vi "Measure vs B2Dv13.vi"() -> ()   [LabVIEW 2009]
doc: "This VI is an example operator panel.\n\nThe VI contains a table for the field values that may be configured manually, or loaded by checking the \"Prompt for File\" box. The data file should contain 3 columns of data, with each column delimited by a tab character.\n\nBefore the VI is executed, set the desired field units and coordinate system. Once the VI is started, follow the directions in the STATUS indicator to operate. Once a field value is achieved, it will be held indefinitely with no user intervention.\n\nThe present field is displayed in the selected units and coordinate system. The present field is queried once per second.\n\nIf a field point is specified that is outside the limits for the magnet, the VI will abort execution."
uses:
  <vilib>/Utility/file.llb/Read From Spreadsheet File (DBL).vi
panel:
  in  "TempSensor":bool
  in  "go to zero at end of measurement":bool=TRUE
  in  "AH (2500)":bool=TRUE
  out "fieldvalues":string[](array[string])
  in  "Nr. of Accumulations":i32=3
  out "appended array":dbl[](array[numeric])=[0.9997924469608681, 60.08772171794918, 0.0, 0.0, 0.0, 0.0, 0.0, 0.0, 0.0, 0.0, 0.0, 1.3266266666666666, -0.0011233333333333334, 0.0, 3432145944.794314]
  in  "X Axis":enum16{"B", "phi"}(ring)=enum."phi"
  in  "Y Axis":T1(ring)=enum."AH C (pF)"
  out "XY Graph":T2(graph)
  in  "GPIB HP 2":string="13"
  in  "Wait between \nVectors":bool=TRUE
  in  "Change\nPID\n(polar coordinates)":bool
  in  "Wait between \nVectors (ms)":u32=2000
  out "measured data":dbl[][](array[numeric])
  in  "Notes:":string="Datum: 3.10.12, Uhrzeit: 19:45, Sweep 0.15T/min,(measurevsB2Dv13.vi)), kapazitive Messung, Probe MnSi 10nm auf CuBe Cantilever (SI078)  tmeasure=ca. 4.3K,,   Einbauwinkel 15° (PraktikumsProbenstab) ,average time 3, winkelsweep mit0.5deg, Messbrücke auf Regal gestellt" caption="Notizen:"
  out "Messfile Refnum":refnum<file>
  in  "Measurement File":path=path "D:/UserData/Matthias/Messungen/MnSi/121003/SI078_121003_4K_m1.txt"
  in  "Sample name:":string="SI078"
  in  "HP 1":bool
  in  "GPIB HP":string="14"
  in  "HP 2":bool
  in  "LI 3":bool
  in  "GPIB L 3":string="8"
  in  "LI 2":bool
  in  "GPIB L 2":string="8"
  in  "LI 1":bool
  in  "GPIB L 1":string="8"
  out "Number of lines":i32=1804
  in  "Operation":u16(ring)=1 items=["Stepwise", "Continous"]
  out "Ramp Rate along Vector (T/min)":dbl=0.15 format="%.3f"
  out "Current Ramp Rate Z (T/min)":dbl=0.1299012842990965 format="%.3f"
  out "Current Ramp Rate Y (T/min)":dbl=0.07500437545533797 format="%.3f"
  in  "User defined Ramp Rate (T/min)":bool=TRUE
  in  "User defined Ramp Rate (T/min)":dbl=0.15 format="%.3f"
  in  "Z-Axis Communications Config":T3={"GPIB address"=22, "GPIB bus"=1, "connection ID"=refnum, "IP"="111.111.111.1", "Active Comm Interface"=0, "Serial Port"="", "Programmer Type"=0} {"Programmer Type" items=["Model 430", "Model 420"]; "Active Comm Interface" items=["TCP/IP (Model 430 Only)", "RS232", "IEEE488"]}
  in  "Max Ramp Rate - Y Axis (A/s)":dbl=0.055 format="%.3f"
  in  "Max Ramp Rate - Z Axis (A/s)":dbl=0.19 format="%.3f"
  in  "Magnitude Limit (kG)":dbl=45.1 format="%.3f"
  in  "Y-Axis Communications Config":T3={"GPIB address"=22, "GPIB bus"=1, "connection ID"=refnum, "IP"="111.111.111.2", "Active Comm Interface"=0, "Serial Port"="", "Programmer Type"=0} {"Programmer Type" items=["Model 430", "Model 420"]; "Active Comm Interface" items=["TCP/IP (Model 430 Only)", "RS232", "IEEE488"]}
  out "Cartesian Display (T)":T4={"Y-Axis Field (T)"=0.01746, "Z-Axis Field (T)"=0.99986} {"Z-Axis Field (T)" format="%.3f"; "Y-Axis Field (T)" format="%.3f"}
  in  "Starting index":i32=1804
  in  "Normal color":u32(colorbox)=11711154
  in  "Highlight color":u32(colorbox)=16711680
  in  "Prompt for File?":bool=TRUE
  out "Continue Execution?":bool
  out "error out":T5
  in  "error in":T5
  out "STATUS":string="Holding at current vector. Set Ramping Mode to NEXT VECTOR to continue."
  in  "Ramping Control":u16(ring)=2 items=["NEXT VECTOR", "RAMPING", "HOLDING", "PAUSE", "ZERO"]
  out "Cartesian Display (kG)":T6 {"Z-Axis Field (kG)" format="%.3f"; "Y-Axis Field (kG)" format="%.3f"}
  in  "Field Values":string[][](table)=[["0.0000", "60.0000"], ["0.3000", "60.0000"], ["0.3000", "60.5000"], ["0.3000", "61.0000"], ["0.3000", "61.5000"], ["0.3000", "62.0000"], ["0.3000", "62.5000"], ["0.3000", "63.0000"], ["0.3000", "63.5000"], ["0.3000", "64.0000"], ["0.3000", "64.5000"], ["0.3000", "65.0000"], ["0.3000", "65.5000"], ["0.3000", "66.0000"], ["0.3000", "66.5000"], ["0.3000", "67.0000"], ["0.3000", "67.5000"], ["0.3000", "68.0000"], ["0.3000", "68.5000"], ["0.3000", "69.0000"], ["0.3000", "69.5000"], ["0.3000", "70.0000"], ["0.3000", "70.5000"], ["0.3000", "71.0000"], ["0.3000", "71.5000"], ["0.3000", "72.0000"], ["0.3000", "72.5000"], ["0.3000", "73.0000"], ["0.3000", "73.5000"], ["0.3000", "74.0000"], ["0.3000", "74.5000"], ["0.3000", "75.0000"], ["0.3000", "75.5000"], ["0.3000", "76.0000"], ["0.3000", "76.5000"], ["0.3000", "77.0000"], ["0.3000", "77.5000"], ["0.3000", "78.0000"], ["0.3000", "78.5000"], ["0.3000", "79.0000"], ["0.3000", "79.5000"], ["0.3000", "80.0000"], ["0.3000", "80.5000"], ["0.3000", "81.0000"], ["0.3000", "81.5000"], ["0.3000", "82.0000"], ["0.3000", "82.5000"], ["0.3000", "83.0000"], ["0.3000", "83.5000"], ["0.3000", "84.0000"], ["0.3000", "84.5000"], ["0.3000", "85.0000"], ["0.3000", "85.5000"], ["0.3000", "86.0000"], ["0.3000", "86.5000"], ["0.3000", "87.0000"], ["0.3000", "87.5000"], ["0.3000", "88.0000"], ["0.3000", "88.5000"], ["0.3000", "89.0000"], ["0.3000", "89.5000"], ["0.3000", "90.0000"], ["0.3000", "90.5000"], ["0.3000", "91.0000"], ["0.3000", "91.5000"], ["0.3000", "92.0000"], ["0.3000", "92.5000"], ["0.3000", "93.0000"], ["0.3000", "93.5000"], ["0.3000", "94.0000"], ["0.3000", "94.5000"], ["0.3000", "95.0000"], ["0.3000", "95.5000"], ["0.3000", "96.0000"], ["0.3000", "96.5000"], ["0.3000", "97.0000"], ["0.3000", "97.5000"], ["0.3000", "98.0000"], ["0.3000", "98.5000"], ["0.3000", "99.0000"], ["0.3000", "99.5000"], ["0.3000", "100.0000"], ["0.3000", "100.5000"], ["0.3000", "101.0000"], ["0.3000", "101.5000"], ["0.3000", "102.0000"], ["0.3000", "102.5000"], ["0.3000", "103.0000"], ["0.3000", "103.5000"], ["0.3000", "104.0000"], ["0.3000", "104.5000"], ["0.3000", "105.0000"], ["0.3000", "105.5000"], ["0.3000", "106.0000"], ["0.3000", "106.5000"], ["0.3000", "107.0000"], ["0.3000", "107.5000"], ["0.3000", "108.0000"], ["0.3000", "108.5000"], ["0.3000", "109.0000"], ["0.3000", "109.5000"], ["0.3000", "110.0000"], ["0.3000", "110.5000"], ["0.3000", "111.0000"], ["0.3000", "111.5000"], ["0.3000", "112.0000"], ["0.3000", "112.5000"], ["0.3000", "113.0000"], ["0.3000", "113.5000"], ["0.3000", "114.0000"], ["0.3000", "114.5000"], ["0.3000", "115.0000"], ["0.3000", "115.5000"], ["0.3000", "116.0000"], ["0.3000", "116.5000"], ["0.3000", "117.0000"], ["0.3000", "117.5000"], ["0.3000", "118.0000"], ["0.3000", "118.5000"], ["0.3000", "119.0000"], ["0.3000", "119.5000"], ["0.3000", "120.0000"], ["0.3000", "120.5000"], ["0.3000", "121.0000"], ["0.3000", "121.5000"], ["0.3000", "122.0000"], ["0.3000", "122.5000"], ["0.3000", "123.0000"], ["0.3000", "123.5000"], ["0.3000", "124.0000"], ["0.3000", "124.5000"], ["0.3000", "125.0000"], ["0.3000", "125.5000"], ["0.3000", "126.0000"], ["0.3000", "126.5000"], ["0.3000", "127.0000"], ["0.3000", "127.5000"], ["0.3000", "128.0000"], ["0.3000", "128.5000"], ["0.3000", "129.0000"], ["0.3000", "129.5000"], ["0.3000", "130.0000"], ["0.3000", "130.5000"], ["0.3000", "131.0000"], ["0.3000", "131.5000"], ["0.3000", "132.0000"], ["0.3000", "132.5000"], ["0.3000", "133.0000"], ["0.3000", "133.5000"], ["0.3000", "134.0000"], ["0.3000", "134.5000"], ["0.3000", "135.0000"], ["0.3000", "135.5000"], ["0.3000", "136.0000"], ["0.3000", "136.5000"], ["0.3000", "137.0000"], ["0.3000", "137.5000"], ["0.3000", "138.0000"], ["0.3000", "138.5000"], ["0.3000", "139.0000"], ["0.3000", "139.5000"], ["0.3000", "140.0000"], ["0.3000", "140.5000"], ["0.3000", "141.0000"], ["0.3000", "141.5000"], ["0.3000", "142.0000"], ["0.3000", "142.5000"], ["0.3000", "143.0000"], ["0.3000", "143.5000"], ["0.3000", "144.0000"], ["0.3000", "144.5000"], ["0.3000", "145.0000"], ["0.3000", "145.5000"], ["0.3000", "146.0000"], ["0.3000", "146.5000"], ["0.3000", "147.0000"], ["0.3000", "147.5000"], ["0.3000", "148.0000"], ["0.3000", "148.5000"], ["0.3000", "149.0000"], ["0.3000", "149.5000"], ["0.3000", "150.0000"], ["0.3000", "150.5000"], ["0.3000", "151.0000"], ["0.3000", "151.5000"], ["0.3000", "152.0000"], ["0.3000", "152.5000"], ["0.3000", "153.0000"], ["0.3000", "153.5000"], ["0.3000", "154.0000"], ["0.3000", "154.5000"], ["0.3000", "155.0000"], ["0.3000", "155.5000"], ["0.3000", "156.0000"], ["0.3000", "156.5000"], ["0.3000", "157.0000"], ["0.3000", "157.5000"], ["0.3000", "158.0000"], ["0.3000", "158.5000"], ["0.3000", "159.0000"], ["0.3000", "159.5000"], ["0.3000", "160.0000"], ["0.3000", "160.5000"], ["0.3000", "161.0000"], ["0.3000", "161.5000"], ["0.3000", "162.0000"], ["0.3000", "162.5000"], ["0.3000", "163.0000"], ["0.3000", "163.5000"], ["0.3000", "164.0000"], ["0.3000", "164.5000"], ["0.3000", "165.0000"], ["0.3000", "165.5000"], ["0.3000", "166.0000"], ["0.3000", "166.5000"], ["0.3000", "167.0000"], ["0.3000", "167.5000"], ["0.3000", "168.0000"], ["0.3000", "168.5000"], ["0.3000", "169.0000"], ["0.3000", "169.5000"], ["0.3000", "170.0000"], ["0.3000", "170.5000"], ["0.3000", "171.0000"], ["0.3000", "171.5000"], ["0.3000", "172.0000"], ["0.3000", "172.5000"], ["0.3000", "173.0000"], ["0.3000", "173.5000"], ["0.3000", "174.0000"], ["0.3000", "174.5000"], ["0.3000", "175.0000"], ["0.3000", "175.5000"], ["0.3000", "176.0000"], ["0.3000", "176.5000"], ["0.3000", "177.0000"], ["0.3000", "177.5000"], ["0.3000", "178.0000"], ["0.3000", "178.5000"], ["0.3000", "179.0000"], ["0.3000", "179.5000"], ["0.3000", "180.0000"], ["0.3000", "180.5000"], ["0.3000", "181.0000"], ["0.3000", "181.5000"], ["0.3000", "182.0000"], ["0.3000", "182.5000"], ["0.3000", "183.0000"], ["0.3000", "183.5000"], ["0.3000", "184.0000"], ["0.3000", "184.5000"], ["0.3000", "185.0000"], ["0.3000", "185.5000"], ["0.3000", "186.0000"], ["0.3000", "186.5000"], ["0.3000", "187.0000"], ["0.3000", "187.5000"], ["0.3000", "188.0000"], ["0.3000", "188.5000"], ["0.3000", "189.0000"], ["0.3000", "189.5000"], ["0.3000", "190.0000"], ["0.3000", "190.5000"], ["0.3000", "191.0000"], ["0.3000", "191.5000"], ["0.3000", "192.0000"], ["0.3000", "192.5000"], ["0.3000", "193.0000"], ["0.3000", "193.5000"], ["0.3000", "194.0000"], ["0.3000", "194.5000"], ["0.3000", "195.0000"], ["0.3000", "195.5000"], ["0.3000", "196.0000"], ["0.3000", "196.5000"], ["0.3000", "197.0000"], ["0.3000", "197.5000"], ["0.3000", "198.0000"], ["0.3000", "198.5000"], ["0.3000", "199.0000"], ["0.3000", "199.5000"], ["0.3000", "200.0000"], ["0.3000", "200.5000"], ["0.3000", "201.0000"], ["0.3000", "201.5000"], ["0.3000", "202.0000"], ["0.3000", "202.5000"], ["0.3000", "203.0000"], ["0.3000", "203.5000"], ["0.3000", "204.0000"], ["0.3000", "204.5000"], ["0.3000", "205.0000"], ["0.3000", "205.5000"], ["0.3000", "206.0000"], ["0.3000", "206.5000"], ["0.3000", "207.0000"], ["0.3000", "207.5000"], ["0.3000", "208.0000"], ["0.3000", "208.5000"], ["0.3000", "209.0000"], ["0.3000", "209.5000"], ["0.3000", "210.0000"], ["0.3000", "210.5000"], ["0.3000", "211.0000"], ["0.3000", "211.5000"], ["0.3000", "212.0000"], ["0.3000", "212.5000"], ["0.3000", "213.0000"], ["0.3000", "213.5000"], ["0.3000", "214.0000"], ["0.3000", "214.5000"], ["0.3000", "215.0000"], ["0.3000", "215.5000"], ["0.3000", "216.0000"], ["0.3000", "216.5000"], ["0.3000", "217.0000"], ["0.3000", "217.5000"], ["0.3000", "218.0000"], ["0.3000", "218.5000"], ["0.3000", "219.0000"], ["0.3000", "219.5000"], ["0.3000", "220.0000"], ["0.3000", "220.5000"], ["0.3000", "221.0000"], ["0.3000", "221.5000"], ["0.3000", "222.0000"], ["0.3000", "222.5000"], ["0.3000", "223.0000"], ["0.3000", "223.5000"], ["0.3000", "224.0000"], ["0.3000", "224.5000"], ["0.3000", "225.0000"], ["0.3000", "225.5000"], ["0.3000", "226.0000"], ["0.3000", "226.5000"], ["0.3000", "227.0000"], ["0.3000", "227.5000"], ["0.3000", "228.0000"], ["0.3000", "228.5000"], ["0.3000", "229.0000"], ["0.3000", "229.5000"], ["0.3000", "230.0000"], ["0.3000", "230.5000"], ["0.3000", "231.0000"], ["0.3000", "231.5000"], ["0.3000", "232.0000"], ["0.3000", "232.5000"], ["0.3000", "233.0000"], ["0.3000", "233.5000"], ["0.3000", "234.0000"], ["0.3000", "234.5000"], ["0.3000", "235.0000"], ["0.3000", "235.5000"], ["0.3000", "236.0000"], ["0.3000", "236.5000"], ["0.3000", "237.0000"], ["0.3000", "237.5000"], ["0.3000", "238.0000"], ["0.3000", "238.5000"], ["0.3000", "239.0000"], ["0.3000", "239.5000"], ["0.3000", "240.0000"], ["0.3000", "240.5000"], ["0.3000", "241.0000"], ["0.3000", "241.5000"], ["0.3000", "242.0000"], ["0.3000", "242.5000"], ["0.3000", "243.0000"], ["0.3000", "243.5000"], ["0.3000", "244.0000"], ["0.3000", "244.5000"], ["0.3000", "245.0000"], ["0.3000", "245.5000"], ["0.3000", "246.0000"], ["0.3000", "246.5000"], ["0.3000", "247.0000"], ["0.3000", "247.5000"], ["0.3000", "248.0000"], ["0.3000", "248.5000"], ["0.3000", "249.0000"], ["0.3000", "249.5000"], ["0.3000", "250.0000"], ["0.3000", "250.5000"], ["0.3000", "251.0000"], ["0.3000", "251.5000"], ["0.3000", "252.0000"], ["0.3000", "252.5000"], ["0.3000", "253.0000"], ["0.3000", "253.5000"], ["0.3000", "254.0000"], ["0.3000", "254.5000"], ["0.3000", "255.0000"], ["0.3000", "255.5000"], ["0.3000", "256.0000"], ["0.3000", "256.5000"], ["0.3000", "257.0000"], ["0.3000", "257.5000"], ["0.3000", "258.0000"], ["0.3000", "258.5000"], ["0.3000", "259.0000"], ["0.3000", "259.5000"], ["0.3000", "260.0000"], ["0.3000", "260.5000"], ["0.3000", "261.0000"], ["0.3000", "261.5000"], ["0.3000", "262.0000"], ["0.3000", "262.5000"], ["0.3000", "263.0000"], ["0.3000", "263.5000"], ["0.3000", "264.0000"], ["0.3000", "264.5000"], ["0.3000", "265.0000"], ["0.3000", "265.5000"], ["0.3000", "266.0000"], ["0.3000", "266.5000"], ["0.3000", "267.0000"], ["0.3000", "267.5000"], ["0.3000", "268.0000"], ["0.3000", "268.5000"], ["0.3000", "269.0000"], ["0.3000", "269.5000"], ["0.3000", "270.0000"], ["0.3000", "270.5000"], ["0.3000", "271.0000"], ["0.3000", "271.5000"], ["0.3000", "272.0000"], ["0.3000", "272.5000"], ["0.3000", "273.0000"], ["0.3000", "273.5000"], ["0.3000", "274.0000"], ["0.3000", "274.5000"], ["0.3000", "275.0000"], ["0.3000", "275.5000"], ["0.3000", "276.0000"], ["0.3000", "276.5000"], ["0.3000", "277.0000"], ["0.3000", "277.5000"], ["0.3000", "278.0000"], ["0.3000", "278.5000"], ["0.3000", "279.0000"], ["0.3000", "279.5000"], ["0.3000", "280.0000"], ["0.3000", "280.5000"], ["0.3000", "281.0000"], ["0.3000", "281.5000"], ["0.3000", "282.0000"], ["0.3000", "282.5000"], ["0.3000", "283.0000"], ["0.3000", "283.5000"], ["0.3000", "284.0000"], ["0.3000", "284.5000"], ["0.3000", "285.0000"], ["0.3000", "284.5000"], ["0.3000", "284.0000"], ["0.3000", "283.5000"], ["0.3000", "283.0000"], ["0.3000", "282.5000"], ["0.3000", "282.0000"], ["0.3000", "281.5000"], ["0.3000", "281.0000"], ["0.3000", "280.5000"], ["0.3000", "280.0000"], ["0.3000", "279.5000"], ["0.3000", "279.0000"], ["0.3000", "278.5000"], ["0.3000", "278.0000"], ["0.3000", "277.5000"], ["0.3000", "277.0000"], ["0.3000", "276.5000"], ["0.3000", "276.0000"], ["0.3000", "275.5000"], ["0.3000", "275.0000"], ["0.3000", "274.5000"], ["0.3000", "274.0000"], ["0.3000", "273.5000"], ["0.3000", "273.0000"], ["0.3000", "272.5000"], ["0.3000", "272.0000"], ["0.3000", "271.5000"], ["0.3000", "271.0000"], ["0.3000", "270.5000"], ["0.3000", "270.0000"], ["0.3000", "269.5000"], ["0.3000", "269.0000"], ["0.3000", "268.5000"], ["0.3000", "268.0000"], ["0.3000", "267.5000"], ["0.3000", "267.0000"], ["0.3000", "266.5000"], ["0.3000", "266.0000"], ["0.3000", "265.5000"], ["0.3000", "265.0000"], ["0.3000", "264.5000"], ["0.3000", "264.0000"], ["0.3000", "263.5000"], ["0.3000", "263.0000"], ["0.3000", "262.5000"], ["0.3000", "262.0000"], ["0.3000", "261.5000"], ["0.3000", "261.0000"], ["0.3000", "260.5000"], ["0.3000", "260.0000"], ["0.3000", "259.5000"], ["0.3000", "259.0000"], ["0.3000", "258.5000"], ["0.3000", "258.0000"], ["0.3000", "257.5000"], ["0.3000", "257.0000"], ["0.3000", "256.5000"], ["0.3000", "256.0000"], ["0.3000", "255.5000"], ["0.3000", "255.0000"], ["0.3000", "254.5000"], ["0.3000", "254.0000"], ["0.3000", "253.5000"], ["0.3000", "253.0000"], ["0.3000", "252.5000"], ["0.3000", "252.0000"], ["0.3000", "251.5000"], ["0.3000", "251.0000"], ["0.3000", "250.5000"], ["0.3000", "250.0000"], ["0.3000", "249.5000"], ["0.3000", "249.0000"], ["0.3000", "248.5000"], ["0.3000", "248.0000"], ["0.3000", "247.5000"], ["0.3000", "247.0000"], ["0.3000", "246.5000"], ["0.3000", "246.0000"], ["0.3000", "245.5000"], ["0.3000", "245.0000"], ["0.3000", "244.5000"], ["0.3000", "244.0000"], ["0.3000", "243.5000"], ["0.3000", "243.0000"], ["0.3000", "242.5000"], ["0.3000", "242.0000"], ["0.3000", "241.5000"], ["0.3000", "241.0000"], ["0.3000", "240.5000"], ["0.3000", "240.0000"], ["0.3000", "239.5000"], ["0.3000", "239.0000"], ["0.3000", "238.5000"], ["0.3000", "238.0000"], ["0.3000", "237.5000"], ["0.3000", "237.0000"], ["0.3000", "236.5000"], ["0.3000", "236.0000"], ["0.3000", "235.5000"], ["0.3000", "235.0000"], ["0.3000", "234.5000"], ["0.3000", "234.0000"], ["0.3000", "233.5000"], ["0.3000", "233.0000"], ["0.3000", "232.5000"], ["0.3000", "232.0000"], ["0.3000", "231.5000"], ["0.3000", "231.0000"], ["0.3000", "230.5000"], ["0.3000", "230.0000"], ["0.3000", "229.5000"], ["0.3000", "229.0000"], ["0.3000", "228.5000"], ["0.3000", "228.0000"], ["0.3000", "227.5000"], ["0.3000", "227.0000"], ["0.3000", "226.5000"], ["0.3000", "226.0000"], ["0.3000", "225.5000"], ["0.3000", "225.0000"], ["0.3000", "224.5000"], ["0.3000", "224.0000"], ["0.3000", "223.5000"], ["0.3000", "223.0000"], ["0.3000", "222.5000"], ["0.3000", "222.0000"], ["0.3000", "221.5000"], ["0.3000", "221.0000"], ["0.3000", "220.5000"], ["0.3000", "220.0000"], ["0.3000", "219.5000"], ["0.3000", "219.0000"], ["0.3000", "218.5000"], ["0.3000", "218.0000"], ["0.3000", "217.5000"], ["0.3000", "217.0000"], ["0.3000", "216.5000"], ["0.3000", "216.0000"], ["0.3000", "215.5000"], ["0.3000", "215.0000"], ["0.3000", "214.5000"], ["0.3000", "214.0000"], ["0.3000", "213.5000"], ["0.3000", "213.0000"], ["0.3000", "212.5000"], ["0.3000", "212.0000"], ["0.3000", "211.5000"], ["0.3000", "211.0000"], ["0.3000", "210.5000"], ["0.3000", "210.0000"], ["0.3000", "209.5000"], ["0.3000", "209.0000"], ["0.3000", "208.5000"], ["0.3000", "208.0000"], ["0.3000", "207.5000"], ["0.3000", "207.0000"], ["0.3000", "206.5000"], ["0.3000", "206.0000"], ["0.3000", "205.5000"], ["0.3000", "205.0000"], ["0.3000", "204.5000"], ["0.3000", "204.0000"], ["0.3000", "203.5000"], ["0.3000", "203.0000"], ["0.3000", "202.5000"], ["0.3000", "202.0000"], ["0.3000", "201.5000"], ["0.3000", "201.0000"], ["0.3000", "200.5000"], ["0.3000", "200.0000"], ["0.3000", "199.5000"], ["0.3000", "199.0000"], ["0.3000", "198.5000"], ["0.3000", "198.0000"], ["0.3000", "197.5000"], ["0.3000", "197.0000"], ["0.3000", "196.5000"], ["0.3000", "196.0000"], ["0.3000", "195.5000"], ["0.3000", "195.0000"], ["0.3000", "194.5000"], ["0.3000", "194.0000"], ["0.3000", "193.5000"], ["0.3000", "193.0000"], ["0.3000", "192.5000"], ["0.3000", "192.0000"], ["0.3000", "191.5000"], ["0.3000", "191.0000"], ["0.3000", "190.5000"], ["0.3000", "190.0000"], ["0.3000", "189.5000"], ["0.3000", "189.0000"], ["0.3000", "188.5000"], ["0.3000", "188.0000"], ["0.3000", "187.5000"], ["0.3000", "187.0000"], ["0.3000", "186.5000"], ["0.3000", "186.0000"], ["0.3000", "185.5000"], ["0.3000", "185.0000"], ["0.3000", "184.5000"], ["0.3000", "184.0000"], ["0.3000", "183.5000"], ["0.3000", "183.0000"], ["0.3000", "182.5000"], ["0.3000", "182.0000"], ["0.3000", "181.5000"], ["0.3000", "181.0000"], ["0.3000", "180.5000"], ["0.3000", "180.0000"], ["0.3000", "179.5000"], ["0.3000", "179.0000"], ["0.3000", "178.5000"], ["0.3000", "178.0000"], ["0.3000", "177.5000"], ["0.3000", "177.0000"], ["0.3000", "176.5000"], ["0.3000", "176.0000"], ["0.3000", "175.5000"], ["0.3000", "175.0000"], ["0.3000", "174.5000"], ["0.3000", "174.0000"], ["0.3000", "173.5000"], ["0.3000", "173.0000"], ["0.3000", "172.5000"], ["0.3000", "172.0000"], ["0.3000", "171.5000"], ["0.3000", "171.0000"], ["0.3000", "170.5000"], ["0.3000", "170.0000"], ["0.3000", "169.5000"], ["0.3000", "169.0000"], ["0.3000", "168.5000"], ["0.3000", "168.0000"], ["0.3000", "167.5000"], ["0.3000", "167.0000"], ["0.3000", "166.5000"], ["0.3000", "166.0000"], ["0.3000", "165.5000"], ["0.3000", "165.0000"], ["0.3000", "164.5000"], ["0.3000", "164.0000"], ["0.3000", "163.5000"], ["0.3000", "163.0000"], ["0.3000", "162.5000"], ["0.3000", "162.0000"], ["0.3000", "161.5000"], ["0.3000", "161.0000"], ["0.3000", "160.5000"], ["0.3000", "160.0000"], ["0.3000", "159.5000"], ["0.3000", "159.0000"], ["0.3000", "158.5000"], ["0.3000", "158.0000"], ["0.3000", "157.5000"], ["0.3000", "157.0000"], ["0.3000", "156.5000"], ["0.3000", "156.0000"], ["0.3000", "155.5000"], ["0.3000", "155.0000"], ["0.3000", "154.5000"], ["0.3000", "154.0000"], ["0.3000", "153.5000"], ["0.3000", "153.0000"], ["0.3000", "152.5000"], ["0.3000", "152.0000"], ["0.3000", "151.5000"], ["0.3000", "151.0000"], ["0.3000", "150.5000"], ["0.3000", "150.0000"], ["0.3000", "149.5000"], ["0.3000", "149.0000"], ["0.3000", "148.5000"], ["0.3000", "148.0000"], ["0.3000", "147.5000"], ["0.3000", "147.0000"], ["0.3000", "146.5000"], ["0.3000", "146.0000"], ["0.3000", "145.5000"], ["0.3000", "145.0000"], ["0.3000", "144.5000"], ["0.3000", "144.0000"], ["0.3000", "143.5000"], ["0.3000", "143.0000"], ["0.3000", "142.5000"], ["0.3000", "142.0000"], ["0.3000", "141.5000"], ["0.3000", "141.0000"], ["0.3000", "140.5000"], ["0.3000", "140.0000"], ["0.3000", "139.5000"], ["0.3000", "139.0000"], ["0.3000", "138.5000"], ["0.3000", "138.0000"], ["0.3000", "137.5000"], ["0.3000", "137.0000"], ["0.3000", "136.5000"], ["0.3000", "136.0000"], ["0.3000", "135.5000"], ["0.3000", "135.0000"], ["0.3000", "134.5000"], ["0.3000", "134.0000"], ["0.3000", "133.5000"], ["0.3000", "133.0000"], ["0.3000", "132.5000"], ["0.3000", "132.0000"], ["0.3000", "131.5000"], ["0.3000", "131.0000"], ["0.3000", "130.5000"], ["0.3000", "130.0000"], ["0.3000", "129.5000"], ["0.3000", "129.0000"], ["0.3000", "128.5000"], ["0.3000", "128.0000"], ["0.3000", "127.5000"], ["0.3000", "127.0000"], ["0.3000", "126.5000"], ["0.3000", "126.0000"], ["0.3000", "125.5000"], ["0.3000", "125.0000"], ["0.3000", "124.5000"], ["0.3000", "124.0000"], ["0.3000", "123.5000"], ["0.3000", "123.0000"], ["0.3000", "122.5000"], ["0.3000", "122.0000"], ["0.3000", "121.5000"], ["0.3000", "121.0000"], ["0.3000", "120.5000"], ["0.3000", "120.0000"], ["0.3000", "119.5000"], ["0.3000", "119.0000"], ["0.3000", "118.5000"], ["0.3000", "118.0000"], ["0.3000", "117.5000"], ["0.3000", "117.0000"], ["0.3000", "116.5000"], ["0.3000", "116.0000"], ["0.3000", "115.5000"], ["0.3000", "115.0000"], ["0.3000", "114.5000"], ["0.3000", "114.0000"], ["0.3000", "113.5000"], ["0.3000", "113.0000"], ["0.3000", "112.5000"], ["0.3000", "112.0000"], ["0.3000", "111.5000"], ["0.3000", "111.0000"], ["0.3000", "110.5000"], ["0.3000", "110.0000"], ["0.3000", "109.5000"], ["0.3000", "109.0000"], ["0.3000", "108.5000"], ["0.3000", "108.0000"], ["0.3000", "107.5000"], ["0.3000", "107.0000"], ["0.3000", "106.5000"], ["0.3000", "106.0000"], ["0.3000", "105.5000"], ["0.3000", "105.0000"], ["0.3000", "104.5000"], ["0.3000", "104.0000"], ["0.3000", "103.5000"], ["0.3000", "103.0000"], ["0.3000", "102.5000"], ["0.3000", "102.0000"], ["0.3000", "101.5000"], ["0.3000", "101.0000"], ["0.3000", "100.5000"], ["0.3000", "100.0000"], ["0.3000", "99.5000"], ["0.3000", "99.0000"], ["0.3000", "98.5000"], ["0.3000", "98.0000"], ["0.3000", "97.5000"], ["0.3000", "97.0000"], ["0.3000", "96.5000"], ["0.3000", "96.0000"], ["0.3000", "95.5000"], ["0.3000", "95.0000"], ["0.3000", "94.5000"], ["0.3000", "94.0000"], ["0.3000", "93.5000"], ["0.3000", "93.0000"], ["0.3000", "92.5000"], ["0.3000", "92.0000"], ["0.3000", "91.5000"], ["0.3000", "91.0000"], ["0.3000", "90.5000"], ["0.3000", "90.0000"], ["0.3000", "89.5000"], ["0.3000", "89.0000"], ["0.3000", "88.5000"], ["0.3000", "88.0000"], ["0.3000", "87.5000"], ["0.3000", "87.0000"], ["0.3000", "86.5000"], ["0.3000", "86.0000"], ["0.3000", "85.5000"], ["0.3000", "85.0000"], ["0.3000", "84.5000"], ["0.3000", "84.0000"], ["0.3000", "83.5000"], ["0.3000", "83.0000"], ["0.3000", "82.5000"], ["0.3000", "82.0000"], ["0.3000", "81.5000"], ["0.3000", "81.0000"], ["0.3000", "80.5000"], ["0.3000", "80.0000"], ["0.3000", "79.5000"], ["0.3000", "79.0000"], ["0.3000", "78.5000"], ["0.3000", "78.0000"], ["0.3000", "77.5000"], ["0.3000", "77.0000"], ["0.3000", "76.5000"], ["0.3000", "76.0000"], ["0.3000", "75.5000"], ["0.3000", "75.0000"], ["0.3000", "74.5000"], ["0.3000", "74.0000"], ["0.3000", "73.5000"], ["0.3000", "73.0000"], ["0.3000", "72.5000"], ["0.3000", "72.0000"], ["0.3000", "71.5000"], ["0.3000", "71.0000"], ["0.3000", "70.5000"], ["0.3000", "70.0000"], ["0.3000", "69.5000"], ["0.3000", "69.0000"], ["0.3000", "68.5000"], ["0.3000", "68.0000"], ["0.3000", "67.5000"], ["0.3000", "67.0000"], ["0.3000", "66.5000"], ["0.3000", "66.0000"], ["0.3000", "65.5000"], ["0.3000", "65.0000"], ["0.3000", "64.5000"], ["0.3000", "64.0000"], ["0.3000", "63.5000"], ["0.3000", "63.0000"], ["0.3000", "62.5000"], ["0.3000", "62.0000"], ["0.3000", "61.5000"], ["0.3000", "61.0000"], ["0.3000", "60.5000"], ["0.3000", "60.0000"], ["1.0000", "60.0000"], ["1.0000", "60.5000"], ["1.0000", "61.0000"], ["1.0000", "61.5000"], ["1.0000", "62.0000"], ["1.0000", "62.5000"], ["1.0000", "63.0000"], ["1.0000", "63.5000"], ["1.0000", "64.0000"], ["1.0000", "64.5000"], ["1.0000", "65.0000"], ["1.0000", "65.5000"], ["1.0000", "66.0000"], ["1.0000", "66.5000"], ["1.0000", "67.0000"], ["1.0000", "67.5000"], ["1.0000", "68.0000"], ["1.0000", "68.5000"], ["1.0000", "69.0000"], ["1.0000", "69.5000"], ["1.0000", "70.0000"], ["1.0000", "70.5000"], ["1.0000", "71.0000"], ["1.0000", "71.5000"], ["1.0000", "72.0000"], ["1.0000", "72.5000"], ["1.0000", "73.0000"], ["1.0000", "73.5000"], ["1.0000", "74.0000"], ["1.0000", "74.5000"], ["1.0000", "75.0000"], ["1.0000", "75.5000"], ["1.0000", "76.0000"], ["1.0000", "76.5000"], ["1.0000", "77.0000"], ["1.0000", "77.5000"], ["1.0000", "78.0000"], ["1.0000", "78.5000"], ["1.0000", "79.0000"], ["1.0000", "79.5000"], ["1.0000", "80.0000"], ["1.0000", "80.5000"], ["1.0000", "81.0000"], ["1.0000", "81.5000"], ["1.0000", "82.0000"], ["1.0000", "82.5000"], ["1.0000", "83.0000"], ["1.0000", "83.5000"], ["1.0000", "84.0000"], ["1.0000", "84.5000"], ["1.0000", "85.0000"], ["1.0000", "85.5000"], ["1.0000", "86.0000"], ["1.0000", "86.5000"], ["1.0000", "87.0000"], ["1.0000", "87.5000"], ["1.0000", "88.0000"], ["1.0000", "88.5000"], ["1.0000", "89.0000"], ["1.0000", "89.5000"], ["1.0000", "90.0000"], ["1.0000", "90.5000"], ["1.0000", "91.0000"], ["1.0000", "91.5000"], ["1.0000", "92.0000"], ["1.0000", "92.5000"], ["1.0000", "93.0000"], ["1.0000", "93.5000"], ["1.0000", "94.0000"], ["1.0000", "94.5000"], ["1.0000", "95.0000"], ["1.0000", "95.5000"], ["1.0000", "96.0000"], ["1.0000", "96.5000"], ["1.0000", "97.0000"], ["1.0000", "97.5000"], ["1.0000", "98.0000"], ["1.0000", "98.5000"], ["1.0000", "99.0000"], ["1.0000", "99.5000"], ["1.0000", "100.0000"], ["1.0000", "100.5000"], ["1.0000", "101.0000"], ["1.0000", "101.5000"], ["1.0000", "102.0000"], ["1.0000", "102.5000"], ["1.0000", "103.0000"], ["1.0000", "103.5000"], ["1.0000", "104.0000"], ["1.0000", "104.5000"], ["1.0000", "105.0000"], ["1.0000", "105.5000"], ["1.0000", "106.0000"], ["1.0000", "106.5000"], ["1.0000", "107.0000"], ["1.0000", "107.5000"], ["1.0000", "108.0000"], ["1.0000", "108.5000"], ["1.0000", "109.0000"], ["1.0000", "109.5000"], ["1.0000", "110.0000"], ["1.0000", "110.5000"], ["1.0000", "111.0000"], ["1.0000", "111.5000"], ["1.0000", "112.0000"], ["1.0000", "112.5000"], ["1.0000", "113.0000"], ["1.0000", "113.5000"], ["1.0000", "114.0000"], ["1.0000", "114.5000"], ["1.0000", "115.0000"], ["1.0000", "115.5000"], ["1.0000", "116.0000"], ["1.0000", "116.5000"], ["1.0000", "117.0000"], ["1.0000", "117.5000"], ["1.0000", "118.0000"], ["1.0000", "118.5000"], ["1.0000", "119.0000"], ["1.0000", "119.5000"], ["1.0000", "120.0000"], ["1.0000", "120.5000"], ["1.0000", "121.0000"], ["1.0000", "121.5000"], ["1.0000", "122.0000"], ["1.0000", "122.5000"], ["1.0000", "123.0000"], ["1.0000", "123.5000"], ["1.0000", "124.0000"], ["1.0000", "124.5000"], ["1.0000", "125.0000"], ["1.0000", "125.5000"], ["1.0000", "126.0000"], ["1.0000", "126.5000"], ["1.0000", "127.0000"], ["1.0000", "127.5000"], ["1.0000", "128.0000"], ["1.0000", "128.5000"], ["1.0000", "129.0000"], ["1.0000", "129.5000"], ["1.0000", "130.0000"], ["1.0000", "130.5000"], ["1.0000", "131.0000"], ["1.0000", "131.5000"], ["1.0000", "132.0000"], ["1.0000", "132.5000"], ["1.0000", "133.0000"], ["1.0000", "133.5000"], ["1.0000", "134.0000"], ["1.0000", "134.5000"], ["1.0000", "135.0000"], ["1.0000", "135.5000"], ["1.0000", "136.0000"], ["1.0000", "136.5000"], ["1.0000", "137.0000"], ["1.0000", "137.5000"], ["1.0000", "138.0000"], ["1.0000", "138.5000"], ["1.0000", "139.0000"], ["1.0000", "139.5000"], ["1.0000", "140.0000"], ["1.0000", "140.5000"], ["1.0000", "141.0000"], ["1.0000", "141.5000"], ["1.0000", "142.0000"], ["1.0000", "142.5000"], ["1.0000", "143.0000"], ["1.0000", "143.5000"], ["1.0000", "144.0000"], ["1.0000", "144.5000"], ["1.0000", "145.0000"], ["1.0000", "145.5000"], ["1.0000", "146.0000"], ["1.0000", "146.5000"], ["1.0000", "147.0000"], ["1.0000", "147.5000"], ["1.0000", "148.0000"], ["1.0000", "148.5000"], ["1.0000", "149.0000"], ["1.0000", "149.5000"], ["1.0000", "150.0000"], ["1.0000", "150.5000"], ["1.0000", "151.0000"], ["1.0000", "151.5000"], ["1.0000", "152.0000"], ["1.0000", "152.5000"], ["1.0000", "153.0000"], ["1.0000", "153.5000"], ["1.0000", "154.0000"], ["1.0000", "154.5000"], ["1.0000", "155.0000"], ["1.0000", "155.5000"], ["1.0000", "156.0000"], ["1.0000", "156.5000"], ["1.0000", "157.0000"], ["1.0000", "157.5000"], ["1.0000", "158.0000"], ["1.0000", "158.5000"], ["1.0000", "159.0000"], ["1.0000", "159.5000"], ["1.0000", "160.0000"], ["1.0000", "160.5000"], ["1.0000", "161.0000"], ["1.0000", "161.5000"], ["1.0000", "162.0000"], ["1.0000", "162.5000"], ["1.0000", "163.0000"], ["1.0000", "163.5000"], ["1.0000", "164.0000"], ["1.0000", "164.5000"], ["1.0000", "165.0000"], ["1.0000", "165.5000"], ["1.0000", "166.0000"], ["1.0000", "166.5000"], ["1.0000", "167.0000"], ["1.0000", "167.5000"], ["1.0000", "168.0000"], ["1.0000", "168.5000"], ["1.0000", "169.0000"], ["1.0000", "169.5000"], ["1.0000", "170.0000"], ["1.0000", "170.5000"], ["1.0000", "171.0000"], ["1.0000", "171.5000"], ["1.0000", "172.0000"], ["1.0000", "172.5000"], ["1.0000", "173.0000"], ["1.0000", "173.5000"], ["1.0000", "174.0000"], ["1.0000", "174.5000"], ["1.0000", "175.0000"], ["1.0000", "175.5000"], ["1.0000", "176.0000"], ["1.0000", "176.5000"], ["1.0000", "177.0000"], ["1.0000", "177.5000"], ["1.0000", "178.0000"], ["1.0000", "178.5000"], ["1.0000", "179.0000"], ["1.0000", "179.5000"], ["1.0000", "180.0000"], ["1.0000", "180.5000"], ["1.0000", "181.0000"], ["1.0000", "181.5000"], ["1.0000", "182.0000"], ["1.0000", "182.5000"], ["1.0000", "183.0000"], ["1.0000", "183.5000"], ["1.0000", "184.0000"], ["1.0000", "184.5000"], ["1.0000", "185.0000"], ["1.0000", "185.5000"], ["1.0000", "186.0000"], ["1.0000", "186.5000"], ["1.0000", "187.0000"], ["1.0000", "187.5000"], ["1.0000", "188.0000"], ["1.0000", "188.5000"], ["1.0000", "189.0000"], ["1.0000", "189.5000"], ["1.0000", "190.0000"], ["1.0000", "190.5000"], ["1.0000", "191.0000"], ["1.0000", "191.5000"], ["1.0000", "192.0000"], ["1.0000", "192.5000"], ["1.0000", "193.0000"], ["1.0000", "193.5000"], ["1.0000", "194.0000"], ["1.0000", "194.5000"], ["1.0000", "195.0000"], ["1.0000", "195.5000"], ["1.0000", "196.0000"], ["1.0000", "196.5000"], ["1.0000", "197.0000"], ["1.0000", "197.5000"], ["1.0000", "198.0000"], ["1.0000", "198.5000"], ["1.0000", "199.0000"], ["1.0000", "199.5000"], ["1.0000", "200.0000"], ["1.0000", "200.5000"], ["1.0000", "201.0000"], ["1.0000", "201.5000"], ["1.0000", "202.0000"], ["1.0000", "202.5000"], ["1.0000", "203.0000"], ["1.0000", "203.5000"], ["1.0000", "204.0000"], ["1.0000", "204.5000"], ["1.0000", "205.0000"], ["1.0000", "205.5000"], ["1.0000", "206.0000"], ["1.0000", "206.5000"], ["1.0000", "207.0000"], ["1.0000", "207.5000"], ["1.0000", "208.0000"], ["1.0000", "208.5000"], ["1.0000", "209.0000"], ["1.0000", "209.5000"], ["1.0000", "210.0000"], ["1.0000", "210.5000"], ["1.0000", "211.0000"], ["1.0000", "211.5000"], ["1.0000", "212.0000"], ["1.0000", "212.5000"], ["1.0000", "213.0000"], ["1.0000", "213.5000"], ["1.0000", "214.0000"], ["1.0000", "214.5000"], ["1.0000", "215.0000"], ["1.0000", "215.5000"], ["1.0000", "216.0000"], ["1.0000", "216.5000"], ["1.0000", "217.0000"], ["1.0000", "217.5000"], ["1.0000", "218.0000"], ["1.0000", "218.5000"], ["1.0000", "219.0000"], ["1.0000", "219.5000"], ["1.0000", "220.0000"], ["1.0000", "220.5000"], ["1.0000", "221.0000"], ["1.0000", "221.5000"], ["1.0000", "222.0000"], ["1.0000", "222.5000"], ["1.0000", "223.0000"], ["1.0000", "223.5000"], ["1.0000", "224.0000"], ["1.0000", "224.5000"], ["1.0000", "225.0000"], ["1.0000", "225.5000"], ["1.0000", "226.0000"], ["1.0000", "226.5000"], ["1.0000", "227.0000"], ["1.0000", "227.5000"], ["1.0000", "228.0000"], ["1.0000", "228.5000"], ["1.0000", "229.0000"], ["1.0000", "229.5000"], ["1.0000", "230.0000"], ["1.0000", "230.5000"], ["1.0000", "231.0000"], ["1.0000", "231.5000"], ["1.0000", "232.0000"], ["1.0000", "232.5000"], ["1.0000", "233.0000"], ["1.0000", "233.5000"], ["1.0000", "234.0000"], ["1.0000", "234.5000"], ["1.0000", "235.0000"], ["1.0000", "235.5000"], ["1.0000", "236.0000"], ["1.0000", "236.5000"], ["1.0000", "237.0000"], ["1.0000", "237.5000"], ["1.0000", "238.0000"], ["1.0000", "238.5000"], ["1.0000", "239.0000"], ["1.0000", "239.5000"], ["1.0000", "240.0000"], ["1.0000", "240.5000"], ["1.0000", "241.0000"], ["1.0000", "241.5000"], ["1.0000", "242.0000"], ["1.0000", "242.5000"], ["1.0000", "243.0000"], ["1.0000", "243.5000"], ["1.0000", "244.0000"], ["1.0000", "244.5000"], ["1.0000", "245.0000"], ["1.0000", "245.5000"], ["1.0000", "246.0000"], ["1.0000", "246.5000"], ["1.0000", "247.0000"], ["1.0000", "247.5000"], ["1.0000", "248.0000"], ["1.0000", "248.5000"], ["1.0000", "249.0000"], ["1.0000", "249.5000"], ["1.0000", "250.0000"], ["1.0000", "250.5000"], ["1.0000", "251.0000"], ["1.0000", "251.5000"], ["1.0000", "252.0000"], ["1.0000", "252.5000"], ["1.0000", "253.0000"], ["1.0000", "253.5000"], ["1.0000", "254.0000"], ["1.0000", "254.5000"], ["1.0000", "255.0000"], ["1.0000", "255.5000"], ["1.0000", "256.0000"], ["1.0000", "256.5000"], ["1.0000", "257.0000"], ["1.0000", "257.5000"], ["1.0000", "258.0000"], ["1.0000", "258.5000"], ["1.0000", "259.0000"], ["1.0000", "259.5000"], ["1.0000", "260.0000"], ["1.0000", "260.5000"], ["1.0000", "261.0000"], ["1.0000", "261.5000"], ["1.0000", "262.0000"], ["1.0000", "262.5000"], ["1.0000", "263.0000"], ["1.0000", "263.5000"], ["1.0000", "264.0000"], ["1.0000", "264.5000"], ["1.0000", "265.0000"], ["1.0000", "265.5000"], ["1.0000", "266.0000"], ["1.0000", "266.5000"], ["1.0000", "267.0000"], ["1.0000", "267.5000"], ["1.0000", "268.0000"], ["1.0000", "268.5000"], ["1.0000", "269.0000"], ["1.0000", "269.5000"], ["1.0000", "270.0000"], ["1.0000", "270.5000"], ["1.0000", "271.0000"], ["1.0000", "271.5000"], ["1.0000", "272.0000"], ["1.0000", "272.5000"], ["1.0000", "273.0000"], ["1.0000", "273.5000"], ["1.0000", "274.0000"], ["1.0000", "274.5000"], ["1.0000", "275.0000"], ["1.0000", "275.5000"], ["1.0000", "276.0000"], ["1.0000", "276.5000"], ["1.0000", "277.0000"], ["1.0000", "277.5000"], ["1.0000", "278.0000"], ["1.0000", "278.5000"], ["1.0000", "279.0000"], ["1.0000", "279.5000"], ["1.0000", "280.0000"], ["1.0000", "280.5000"], ["1.0000", "281.0000"], ["1.0000", "281.5000"], ["1.0000", "282.0000"], ["1.0000", "282.5000"], ["1.0000", "283.0000"], ["1.0000", "283.5000"], ["1.0000", "284.0000"], ["1.0000", "284.5000"], ["1.0000", "285.0000"], ["1.0000", "284.5000"], ["1.0000", "284.0000"], ["1.0000", "283.5000"], ["1.0000", "283.0000"], ["1.0000", "282.5000"], ["1.0000", "282.0000"], ["1.0000", "281.5000"], ["1.0000", "281.0000"], ["1.0000", "280.5000"], ["1.0000", "280.0000"], ["1.0000", "279.5000"], ["1.0000", "279.0000"], ["1.0000", "278.5000"], ["1.0000", "278.0000"], ["1.0000", "277.5000"], ["1.0000", "277.0000"], ["1.0000", "276.5000"], ["1.0000", "276.0000"], ["1.0000", "275.5000"], ["1.0000", "275.0000"], ["1.0000", "274.5000"], ["1.0000", "274.0000"], ["1.0000", "273.5000"], ["1.0000", "273.0000"], ["1.0000", "272.5000"], ["1.0000", "272.0000"], ["1.0000", "271.5000"], ["1.0000", "271.0000"], ["1.0000", "270.5000"], ["1.0000", "270.0000"], ["1.0000", "269.5000"], ["1.0000", "269.0000"], ["1.0000", "268.5000"], ["1.0000", "268.0000"], ["1.0000", "267.5000"], ["1.0000", "267.0000"], ["1.0000", "266.5000"], ["1.0000", "266.0000"], ["1.0000", "265.5000"], ["1.0000", "265.0000"], ["1.0000", "264.5000"], ["1.0000", "264.0000"], ["1.0000", "263.5000"], ["1.0000", "263.0000"], ["1.0000", "262.5000"], ["1.0000", "262.0000"], ["1.0000", "261.5000"], ["1.0000", "261.0000"], ["1.0000", "260.5000"], ["1.0000", "260.0000"], ["1.0000", "259.5000"], ["1.0000", "259.0000"], ["1.0000", "258.5000"], ["1.0000", "258.0000"], ["1.0000", "257.5000"], ["1.0000", "257.0000"], ["1.0000", "256.5000"], ["1.0000", "256.0000"], ["1.0000", "255.5000"], ["1.0000", "255.0000"], ["1.0000", "254.5000"], ["1.0000", "254.0000"], ["1.0000", "253.5000"], ["1.0000", "253.0000"], ["1.0000", "252.5000"], ["1.0000", "252.0000"], ["1.0000", "251.5000"], ["1.0000", "251.0000"], ["1.0000", "250.5000"], ["1.0000", "250.0000"], ["1.0000", "249.5000"], ["1.0000", "249.0000"], ["1.0000", "248.5000"], ["1.0000", "248.0000"], ["1.0000", "247.5000"], ["1.0000", "247.0000"], ["1.0000", "246.5000"], ["1.0000", "246.0000"], ["1.0000", "245.5000"], ["1.0000", "245.0000"], ["1.0000", "244.5000"], ["1.0000", "244.0000"], ["1.0000", "243.5000"], ["1.0000", "243.0000"], ["1.0000", "242.5000"], ["1.0000", "242.0000"], ["1.0000", "241.5000"], ["1.0000", "241.0000"], ["1.0000", "240.5000"], ["1.0000", "240.0000"], ["1.0000", "239.5000"], ["1.0000", "239.0000"], ["1.0000", "238.5000"], ["1.0000", "238.0000"], ["1.0000", "237.5000"], ["1.0000", "237.0000"], ["1.0000", "236.5000"], ["1.0000", "236.0000"], ["1.0000", "235.5000"], ["1.0000", "235.0000"], ["1.0000", "234.5000"], ["1.0000", "234.0000"], ["1.0000", "233.5000"], ["1.0000", "233.0000"], ["1.0000", "232.5000"], ["1.0000", "232.0000"], ["1.0000", "231.5000"], ["1.0000", "231.0000"], ["1.0000", "230.5000"], ["1.0000", "230.0000"], ["1.0000", "229.5000"], ["1.0000", "229.0000"], ["1.0000", "228.5000"], ["1.0000", "228.0000"], ["1.0000", "227.5000"], ["1.0000", "227.0000"], ["1.0000", "226.5000"], ["1.0000", "226.0000"], ["1.0000", "225.5000"], ["1.0000", "225.0000"], ["1.0000", "224.5000"], ["1.0000", "224.0000"], ["1.0000", "223.5000"], ["1.0000", "223.0000"], ["1.0000", "222.5000"], ["1.0000", "222.0000"], ["1.0000", "221.5000"], ["1.0000", "221.0000"], ["1.0000", "220.5000"], ["1.0000", "220.0000"], ["1.0000", "219.5000"], ["1.0000", "219.0000"], ["1.0000", "218.5000"], ["1.0000", "218.0000"], ["1.0000", "217.5000"], ["1.0000", "217.0000"], ["1.0000", "216.5000"], ["1.0000", "216.0000"], ["1.0000", "215.5000"], ["1.0000", "215.0000"], ["1.0000", "214.5000"], ["1.0000", "214.0000"], ["1.0000", "213.5000"], ["1.0000", "213.0000"], ["1.0000", "212.5000"], ["1.0000", "212.0000"], ["1.0000", "211.5000"], ["1.0000", "211.0000"], ["1.0000", "210.5000"], ["1.0000", "210.0000"], ["1.0000", "209.5000"], ["1.0000", "209.0000"], ["1.0000", "208.5000"], ["1.0000", "208.0000"], ["1.0000", "207.5000"], ["1.0000", "207.0000"], ["1.0000", "206.5000"], ["1.0000", "206.0000"], ["1.0000", "205.5000"], ["1.0000", "205.0000"], ["1.0000", "204.5000"], ["1.0000", "204.0000"], ["1.0000", "203.5000"], ["1.0000", "203.0000"], ["1.0000", "202.5000"], ["1.0000", "202.0000"], ["1.0000", "201.5000"], ["1.0000", "201.0000"], ["1.0000", "200.5000"], ["1.0000", "200.0000"], ["1.0000", "199.5000"], ["1.0000", "199.0000"], ["1.0000", "198.5000"], ["1.0000", "198.0000"], ["1.0000", "197.5000"], ["1.0000", "197.0000"], ["1.0000", "196.5000"], ["1.0000", "196.0000"], ["1.0000", "195.5000"], ["1.0000", "195.0000"], ["1.0000", "194.5000"], ["1.0000", "194.0000"], ["1.0000", "193.5000"], ["1.0000", "193.0000"], ["1.0000", "192.5000"], ["1.0000", "192.0000"], ["1.0000", "191.5000"], ["1.0000", "191.0000"], ["1.0000", "190.5000"], ["1.0000", "190.0000"], ["1.0000", "189.5000"], ["1.0000", "189.0000"], ["1.0000", "188.5000"], ["1.0000", "188.0000"], ["1.0000", "187.5000"], ["1.0000", "187.0000"], ["1.0000", "186.5000"], ["1.0000", "186.0000"], ["1.0000", "185.5000"], ["1.0000", "185.0000"], ["1.0000", "184.5000"], ["1.0000", "184.0000"], ["1.0000", "183.5000"], ["1.0000", "183.0000"], ["1.0000", "182.5000"], ["1.0000", "182.0000"], ["1.0000", "181.5000"], ["1.0000", "181.0000"], ["1.0000", "180.5000"], ["1.0000", "180.0000"], ["1.0000", "179.5000"], ["1.0000", "179.0000"], ["1.0000", "178.5000"], ["1.0000", "178.0000"], ["1.0000", "177.5000"], ["1.0000", "177.0000"], ["1.0000", "176.5000"], ["1.0000", "176.0000"], ["1.0000", "175.5000"], ["1.0000", "175.0000"], ["1.0000", "174.5000"], ["1.0000", "174.0000"], ["1.0000", "173.5000"], ["1.0000", "173.0000"], ["1.0000", "172.5000"], ["1.0000", "172.0000"], ["1.0000", "171.5000"], ["1.0000", "171.0000"], ["1.0000", "170.5000"], ["1.0000", "170.0000"], ["1.0000", "169.5000"], ["1.0000", "169.0000"], ["1.0000", "168.5000"], ["1.0000", "168.0000"], ["1.0000", "167.5000"], ["1.0000", "167.0000"], ["1.0000", "166.5000"], ["1.0000", "166.0000"], ["1.0000", "165.5000"], ["1.0000", "165.0000"], ["1.0000", "164.5000"], ["1.0000", "164.0000"], ["1.0000", "163.5000"], ["1.0000", "163.0000"], ["1.0000", "162.5000"], ["1.0000", "162.0000"], ["1.0000", "161.5000"], ["1.0000", "161.0000"], ["1.0000", "160.5000"], ["1.0000", "160.0000"], ["1.0000", "159.5000"], ["1.0000", "159.0000"], ["1.0000", "158.5000"], ["1.0000", "158.0000"], ["1.0000", "157.5000"], ["1.0000", "157.0000"], ["1.0000", "156.5000"], ["1.0000", "156.0000"], ["1.0000", "155.5000"], ["1.0000", "155.0000"], ["1.0000", "154.5000"], ["1.0000", "154.0000"], ["1.0000", "153.5000"], ["1.0000", "153.0000"], ["1.0000", "152.5000"], ["1.0000", "152.0000"], ["1.0000", "151.5000"], ["1.0000", "151.0000"], ["1.0000", "150.5000"], ["1.0000", "150.0000"], ["1.0000", "149.5000"], ["1.0000", "149.0000"], ["1.0000", "148.5000"], ["1.0000", "148.0000"], ["1.0000", "147.5000"], ["1.0000", "147.0000"], ["1.0000", "146.5000"], ["1.0000", "146.0000"], ["1.0000", "145.5000"], ["1.0000", "145.0000"], ["1.0000", "144.5000"], ["1.0000", "144.0000"], ["1.0000", "143.5000"], ["1.0000", "143.0000"], ["1.0000", "142.5000"], ["1.0000", "142.0000"], ["1.0000", "141.5000"], ["1.0000", "141.0000"], ["1.0000", "140.5000"], ["1.0000", "140.0000"], ["1.0000", "139.5000"], ["1.0000", "139.0000"], ["1.0000", "138.5000"], ["1.0000", "138.0000"], ["1.0000", "137.5000"], ["1.0000", "137.0000"], ["1.0000", "136.5000"], ["1.0000", "136.0000"], ["1.0000", "135.5000"], ["1.0000", "135.0000"], ["1.0000", "134.5000"], ["1.0000", "134.0000"], ["1.0000", "133.5000"], ["1.0000", "133.0000"], ["1.0000", "132.5000"], ["1.0000", "132.0000"], ["1.0000", "131.5000"], ["1.0000", "131.0000"], ["1.0000", "130.5000"], ["1.0000", "130.0000"], ["1.0000", "129.5000"], ["1.0000", "129.0000"], ["1.0000", "128.5000"], ["1.0000", "128.0000"], ["1.0000", "127.5000"], ["1.0000", "127.0000"], ["1.0000", "126.5000"], ["1.0000", "126.0000"], ["1.0000", "125.5000"], ["1.0000", "125.0000"], ["1.0000", "124.5000"], ["1.0000", "124.0000"], ["1.0000", "123.5000"], ["1.0000", "123.0000"], ["1.0000", "122.5000"], ["1.0000", "122.0000"], ["1.0000", "121.5000"], ["1.0000", "121.0000"], ["1.0000", "120.5000"], ["1.0000", "120.0000"], ["1.0000", "119.5000"], ["1.0000", "119.0000"], ["1.0000", "118.5000"], ["1.0000", "118.0000"], ["1.0000", "117.5000"], ["1.0000", "117.0000"], ["1.0000", "116.5000"], ["1.0000", "116.0000"], ["1.0000", "115.5000"], ["1.0000", "115.0000"], ["1.0000", "114.5000"], ["1.0000", "114.0000"], ["1.0000", "113.5000"], ["1.0000", "113.0000"], ["1.0000", "112.5000"], ["1.0000", "112.0000"], ["1.0000", "111.5000"], ["1.0000", "111.0000"], ["1.0000", "110.5000"], ["1.0000", "110.0000"], ["1.0000", "109.5000"], ["1.0000", "109.0000"], ["1.0000", "108.5000"], ["1.0000", "108.0000"], ["1.0000", "107.5000"], ["1.0000", "107.0000"], ["1.0000", "106.5000"], ["1.0000", "106.0000"], ["1.0000", "105.5000"], ["1.0000", "105.0000"], ["1.0000", "104.5000"], ["1.0000", "104.0000"], ["1.0000", "103.5000"], ["1.0000", "103.0000"], ["1.0000", "102.5000"], ["1.0000", "102.0000"], ["1.0000", "101.5000"], ["1.0000", "101.0000"], ["1.0000", "100.5000"], ["1.0000", "100.0000"], ["1.0000", "99.5000"], ["1.0000", "99.0000"], ["1.0000", "98.5000"], ["1.0000", "98.0000"], ["1.0000", "97.5000"], ["1.0000", "97.0000"], ["1.0000", "96.5000"], ["1.0000", "96.0000"], ["1.0000", "95.5000"], ["1.0000", "95.0000"], ["1.0000", "94.5000"], ["1.0000", "94.0000"], ["1.0000", "93.5000"], ["1.0000", "93.0000"], ["1.0000", "92.5000"], ["1.0000", "92.0000"], ["1.0000", "91.5000"], ["1.0000", "91.0000"], ["1.0000", "90.5000"], ["1.0000", "90.0000"], ["1.0000", "89.5000"], ["1.0000", "89.0000"], ["1.0000", "88.5000"], ["1.0000", "88.0000"], ["1.0000", "87.5000"], ["1.0000", "87.0000"], ["1.0000", "86.5000"], ["1.0000", "86.0000"], ["1.0000", "85.5000"], ["1.0000", "85.0000"], ["1.0000", "84.5000"], ["1.0000", "84.0000"], ["1.0000", "83.5000"], ["1.0000", "83.0000"], ["1.0000", "82.5000"], ["1.0000", "82.0000"], ["1.0000", "81.5000"], ["1.0000", "81.0000"], ["1.0000", "80.5000"], ["1.0000", "80.0000"], ["1.0000", "79.5000"], ["1.0000", "79.0000"], ["1.0000", "78.5000"], ["1.0000", "78.0000"], ["1.0000", "77.5000"], ["1.0000", "77.0000"], ["1.0000", "76.5000"], ["1.0000", "76.0000"], ["1.0000", "75.5000"], ["1.0000", "75.0000"], ["1.0000", "74.5000"], ["1.0000", "74.0000"], ["1.0000", "73.5000"], ["1.0000", "73.0000"], ["1.0000", "72.5000"], ["1.0000", "72.0000"], ["1.0000", "71.5000"], ["1.0000", "71.0000"], ["1.0000", "70.5000"], ["1.0000", "70.0000"], ["1.0000", "69.5000"], ["1.0000", "69.0000"], ["1.0000", "68.5000"], ["1.0000", "68.0000"], ["1.0000", "67.5000"], ["1.0000", "67.0000"], ["1.0000", "66.5000"], ["1.0000", "66.0000"], ["1.0000", "65.5000"], ["1.0000", "65.0000"], ["1.0000", "64.5000"], ["1.0000", "64.0000"], ["1.0000", "63.5000"], ["1.0000", "63.0000"], ["1.0000", "62.5000"], ["1.0000", "62.0000"], ["1.0000", "61.5000"], ["1.0000", "61.0000"], ["1.0000", "60.5000"], ["1.0000", "60.0000"], ["0.0000", "60.0000"]]
  out "Switch Heaters":bool=TRUE
  out "Polar Display (T)":T7={"q (degrees)"=59.03624346792648, "Field Magnitude (T)"=0.00011661903789690601} {"Field Magnitude (T)" format="%.3f"; "q (degrees)" format="%.3f"}
  out "Polar Display (kG)":T8 {"Field Magnitude (kG)" format="%.3f"; "q (degrees)" format="%.3f"}
  in  "Coordinate System":u16(ring)=1 items=["Cartesian", "Polar"]
  in  "Magnetic Field Units":u16(ring)=1 items=["kG", "Tesla"]
  # "Punkt für Punkt Messung, gotozero am Ende der Messung und switch heater off"
  # "Measurement Display"
  # "Measurement Settings"
  # "Magnet Settings"
  # "Max Ramp Rate z: 1.27 T/min\nMax Ramp Rate y: 0.17 T/min"
  # "Devices"
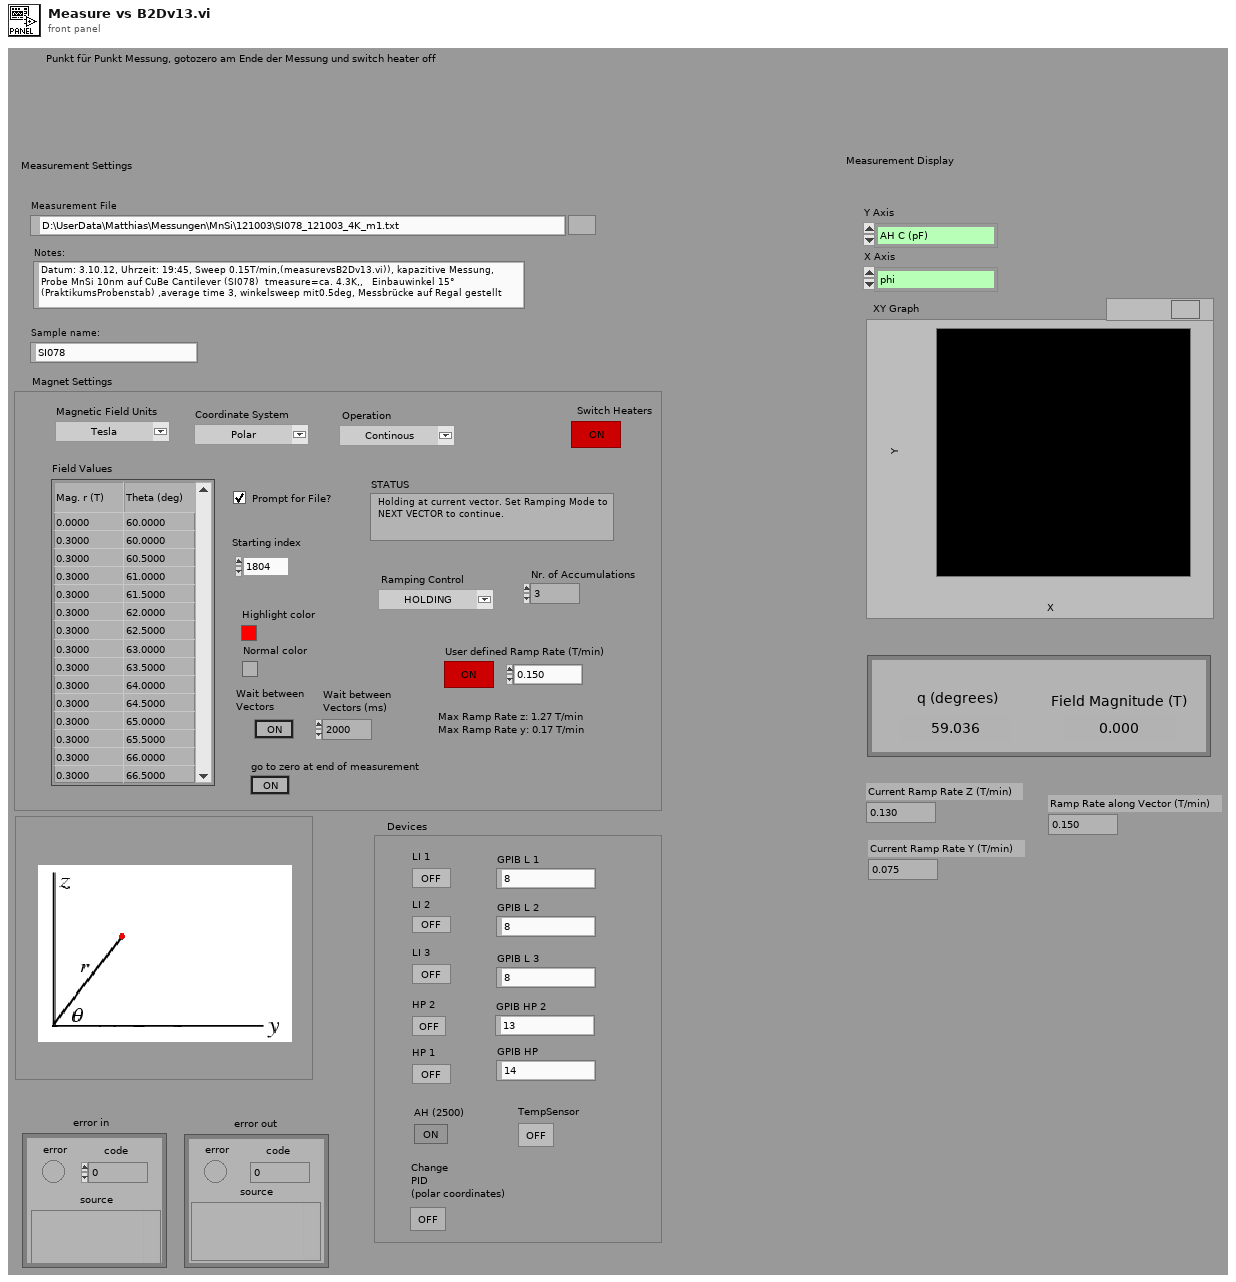
[diagram p1: front panel]
types:
  T1 = enum16{"B", "phi", "LI 1 Vx", "LI 1 phase", "LI 2 Vx", "LI 2 phase", "LI 3 Vx", "LI 3 phase", "LI 4 Vx", "LI 4 phase", "HP (V)", "AH C (pF)", "AH loss", "R Tempsensor"}
  T2 = cluster{"measured data":dbl[], "measured data":dbl[]}
  T3 = cluster{"GPIB address":i16, "GPIB bus":i16, "connection ID":refnum<k5>, "IP":string, "Active Comm Interface":u16, "Serial Port":refnum<visa-resource-name>, "Programmer Type":u16}
  T4 = cluster{"Y-Axis Field (T)":dbl, "Z-Axis Field (T)":dbl}
  T5 = cluster{"error":bool, "code":i32, "source":string}
  T6 = cluster{"Y-Axis Field (kG)":dbl, "Z-Axis Field (kG)":dbl}
  T7 = cluster{"q (degrees)":dbl, "Field Magnitude (T)":dbl}
  T8 = cluster{"q (degrees)":dbl, "Field Magnitude (kG)":dbl}
  T9 = enum16{"", "RAMPING", "HOLDING", "PAUSED", "MANUAL UP", "MANUAL DOWN", "ZEROING CURRENT", "QUENCH DETECTED", "HEATING SWITCH"}
  T10 = enum16{"", "RAMPING", "HOLDING", "PAUSED", "MANUAL UP", "MANUAL DOWN", "ZEROING CURRENT", "QUENCH DETECTED", "HEATING SWITCH", "AT ZER0", "COOLING SWITCH"}
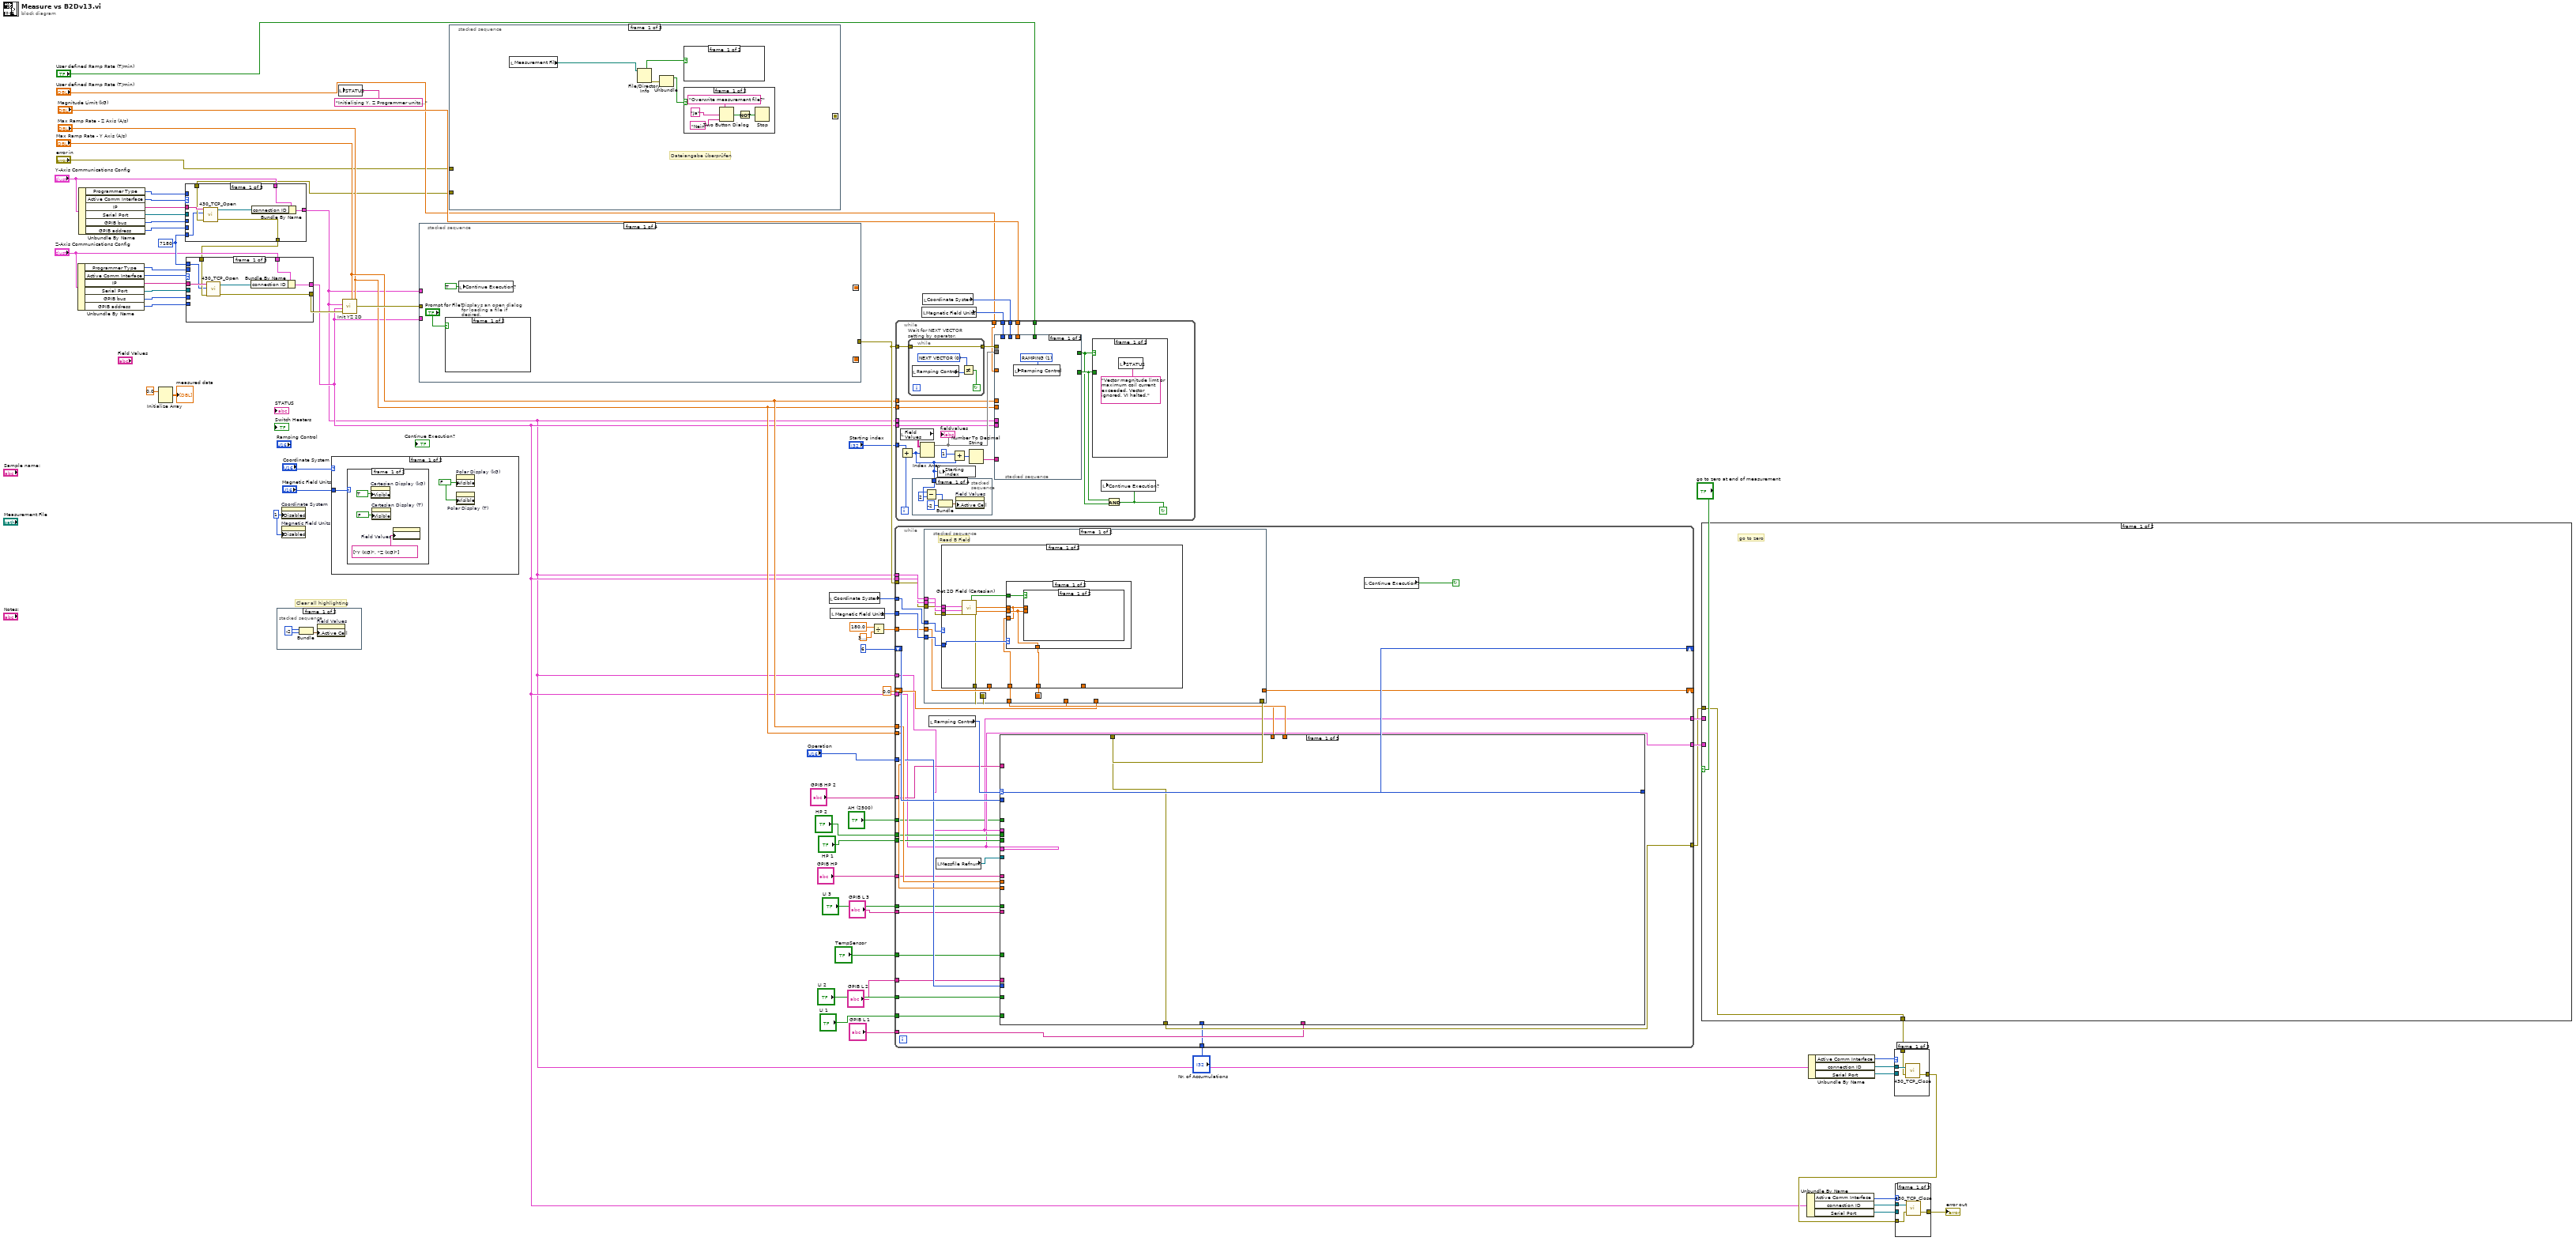
[diagram p0: block diagram]
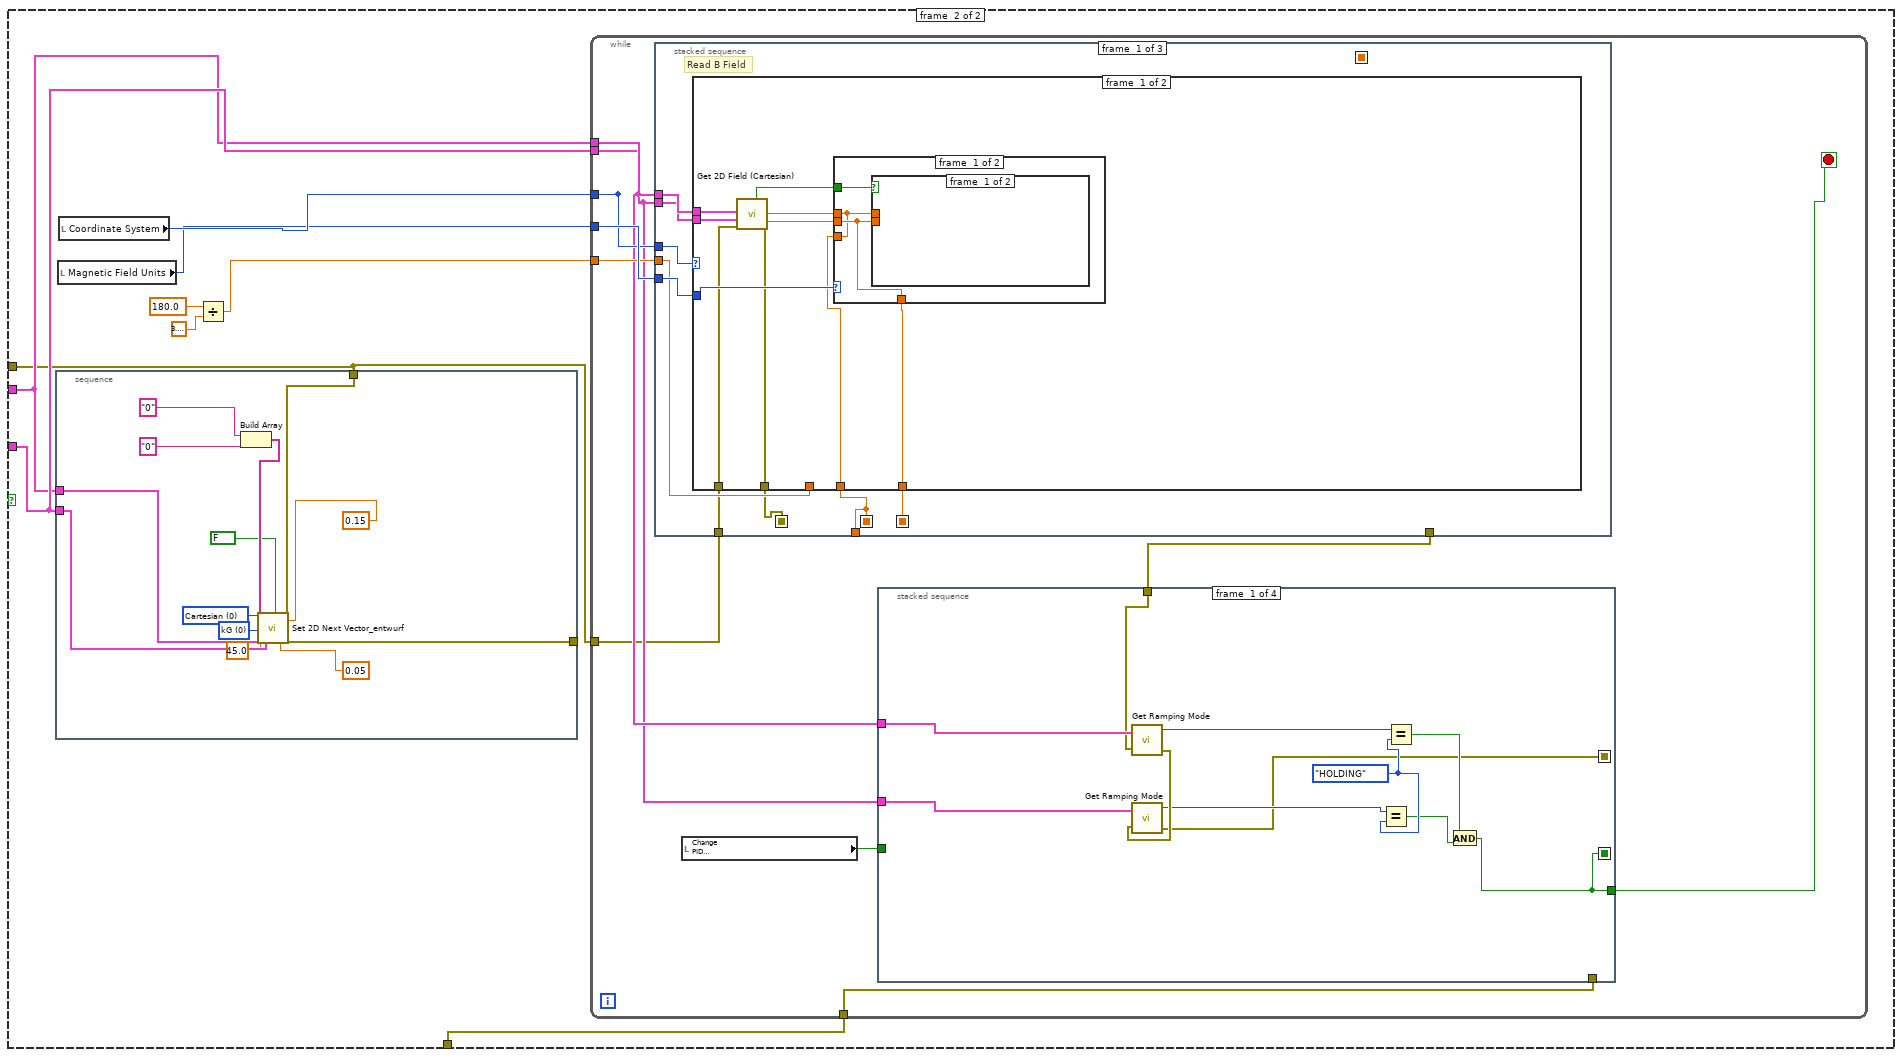
[diagram p2: hidden frame]
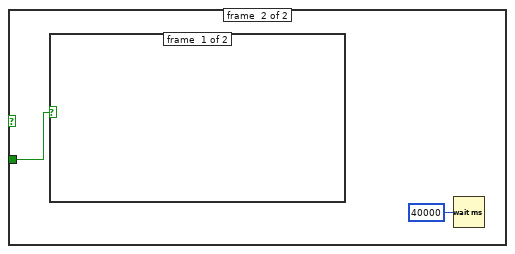
[diagram p4: hidden frame]
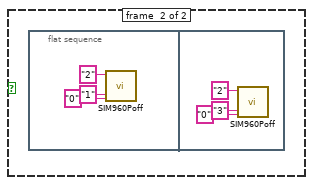
[diagram p5: hidden frame]
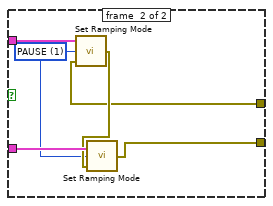
[diagram p7: hidden frame]
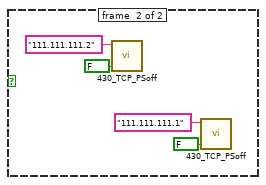
[diagram p9: hidden frame]
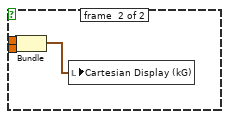
[diagram p10: hidden frame]
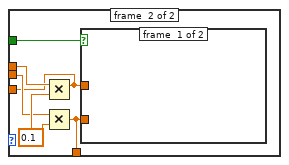
[diagram p11: hidden frame]
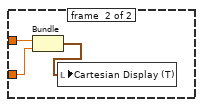
[diagram p12: hidden frame]
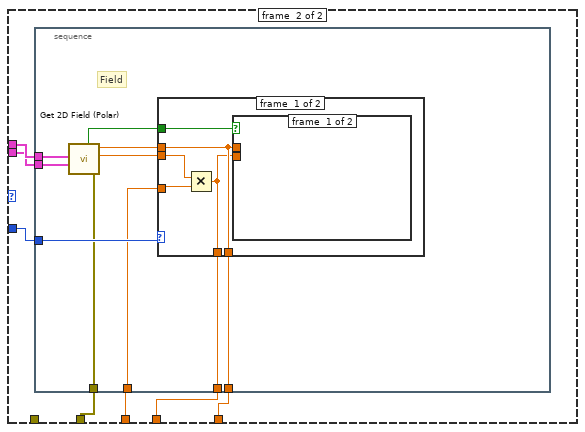
[diagram p13: hidden frame]
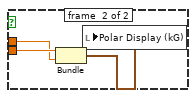
[diagram p14: hidden frame]
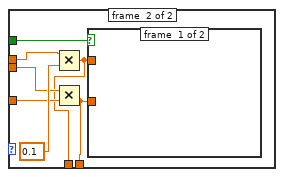
[diagram p15: hidden frame]
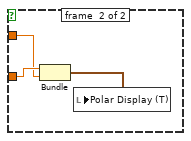
[diagram p16: hidden frame]
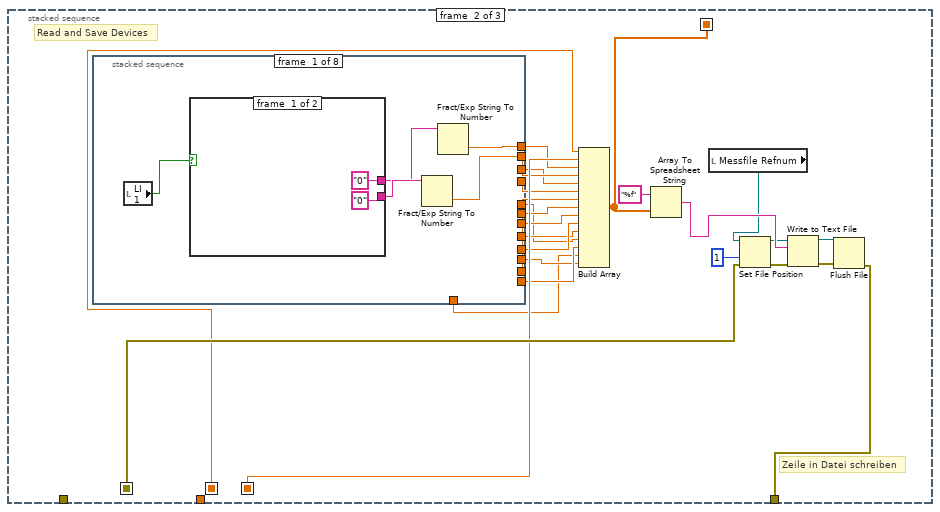
[diagram p17: hidden frame]
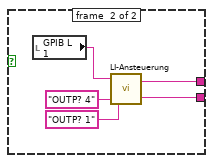
[diagram p18: hidden frame]
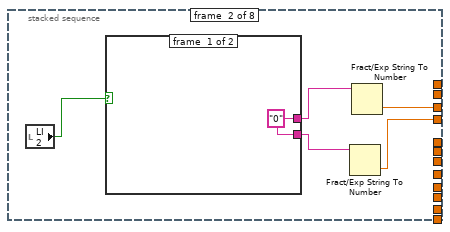
[diagram p19: hidden frame]
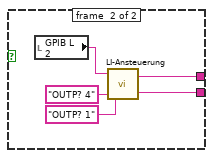
[diagram p20: hidden frame]
diagram:
  w56 = 7180 ("TCP Port")
  w69 = u8 1 ("Write Attribute")
  # "Clear all highlighting"
  n1 = Unbundle By Name("Z-Axis Communications Config") -> ("Programmer Type"=w35:u16, "Active Comm Interface"=w55:u16, "IP"=w52:string, "Serial Port"=w51:refnum<visa-resource-name>, "GPIB bus"=w34:i16, "GPIB address"=w33:i16)
  n2 = Unbundle By Name("Y-Axis Communications Config") -> ("Programmer Type"=w29:u16, "Active Comm Interface"=w54:u16, "IP"=w53:string, "Serial Port"=w50:refnum<visa-resource-name>, "GPIB bus"=w30:i16, "GPIB address"=w31:i16)
  n3 = Initialize Array(0.0 ("element")) -> (→"measured data":dbl[][])  [unwired: 2 in]
  n4 = stacked-sequence {
    frame #0 {
      w72 = -2
      n5 = Bundle(w72, w72) -> (w73:cluster{i32, i32})  [unwired: 1 in]
      n6 = property on="Field Values" class="Tbl (strict)"("Active Cell:Active Cell"=w73) -> ()  [unwired: 2 in, 2 out]
    }
    frame #1 {
      n7 = property on="Field Values" class="Tbl (strict)"("Active Cell:Cell Background Color"="Normal color") -> ()  [unwired: 2 in, 2 out]
    }
  }
  n8 = property on="Coordinate System" class="Ring (strict)"("Disabled"=w69) -> ()  [unwired: 2 in, 2 out]
  n9 = property on="Magnetic Field Units" class="Ring (strict)"("Disabled"=w69) -> ()  [unwired: 2 in, 2 out]
  n10 = case shown="0, Default" "Coordinate System" {
    tunnel: "Magnetic Field Units" -> [w76 w84]
    frame #0 {
      w75 = FALSE ("Write Attribute")
      (unwired) FALSE ("Write Attribute")
      (unwired) TRUE ("Write Attribute")
      n11 = case shown="1" w76 {
        frame #0 {
          n12 = property on="Cartesian Display (kG)" class="Cluster (strict)"("Visible"=TRUE ("Write Attribute")) -> ()  [unwired: 2 in, 2 out]
          n13 = property on="Cartesian Display (T)" class="Cluster (strict)"("Visible"=FALSE ("Write Attribute")) -> ()  [unwired: 2 in, 2 out]
          n14 = property on="Field Values" class="Tbl (strict)"("Column Header Strings[]"=string[] ["Y (KG)", "Z (KG)"] ("Write Attribute")) -> ()  [unwired: 2 in, 2 out]
        }
        frame #1 {
          n15 = property on="Cartesian Display (kG)" class="Cluster (strict)"("Visible"=FALSE ("Write Attribute")) -> ()  [unwired: 2 in, 2 out]
          n16 = property on="Cartesian Display (T)" class="Cluster (strict)"("Visible"=TRUE ("Write Attribute")) -> ()  [unwired: 2 in, 2 out]
          n17 = property on="Field Values" class="Tbl (strict)"("Column Header Strings[]"=string[] ["Y (T)", "Z (T)"] ("Write Attribute")) -> ()  [unwired: 2 in, 2 out]
        }
      }
      n18 = property on="Polar Display (kG)" class="Clust (strict)"("Visible"=w75) -> ()  [unwired: 2 in, 2 out]
      n19 = property on="Polar Display (T)" class="Clust (strict)"("Visible"=w75) -> ()  [unwired: 2 in, 2 out]
    }
    frame #1 {
      (unwired) FALSE ("Write Attribute")
      (unwired) TRUE ("Write Attribute")
      w83 = FALSE ("Write Attribute")
      n20 = case shown="1" w84 {
        frame #0 {
          n21 = property on="Polar Display (kG)" class="Clust (strict)"("Visible"=TRUE ("Write Attribute")) -> ()  [unwired: 2 in, 2 out]
          n22 = property on="Polar Display (T)" class="Clust (strict)"("Visible"=FALSE ("Write Attribute")) -> ()  [unwired: 2 in, 2 out]
          n23 = property on="Field Values" class="Tbl (strict)"("Column Header Strings[]"=string[] ["Mag. r (KG)", "Theta (deg)"] ("Write Attribute")) -> ()  [unwired: 2 in, 2 out]
        }
        frame #1 {
          n24 = property on="Polar Display (kG)" class="Clust (strict)"("Visible"=FALSE ("Write Attribute")) -> ()  [unwired: 2 in, 2 out]
          n25 = property on="Polar Display (T)" class="Clust (strict)"("Visible"=TRUE ("Write Attribute")) -> ()  [unwired: 2 in, 2 out]
          n26 = property on="Field Values" class="Tbl (strict)"("Column Header Strings[]"=string[] ["Mag. r (T)", "Theta (deg)"] ("Write Attribute")) -> ()  [unwired: 2 in, 2 out]
        }
      }
      n27 = property on="Cartesian Display (kG)" class="Cluster (strict)"("Visible"=w83) -> ()  [unwired: 2 in, 2 out]
      n28 = property on="Cartesian Display (T)" class="Cluster (strict)"("Visible"=w83) -> ()  [unwired: 2 in, 2 out]
    }
  }
  n29 = local write "STATUS"("Initializing Y, Z Programmer units..." ("STATUS")) -> ()
  n30 = stacked-sequence {
    seq-local: [_ w102 _] -> [_ _ w127]
    tunnel: "error in" -> [_ w103 _]
    tunnel: [_ _ w126] -> w24
    frame #0 {
      # "Dateiangabe überprüfen"
      n31 = local read "Measurement File"() -> (w94:path)
      n32 = File/Directory Info(path=w94) -> (directory=w92:bool, error out=w93:errorcluster)  [unwired: 1 in, 5 out]
      n33 = Unbundle(w93) -> ("status"=w91:bool)  [unwired: 2 out]
      n34 = case shown="False" w92 {
        frame #0 {
        }
        frame #1 {
          n35 = One Button Dialog(message="Invalid\nfilename!") -> (true=w100:bool)  [unwired: 1 in]
          n36 = Stop(stop? (T)=w100) -> ()
        }
      }
      n37 = case shown="False" w91 {
        frame #0 {
          n38 = Two Button Dialog(message="Overwrite measurement file?", 1:"Nein", 2:"Ja") -> (T button?=w96:bool)
          n39 = Not(x=w96) -> (.not. x?=w95:bool)
          n40 = Stop(stop? (T)=w95) -> ()
        }
        frame #1 {
        }
      }
    }
    frame #1 {
      w106 = "\r"
      # "Erstellen\ndes Headers"
      n41 = local read "User defined Ramp Rate (T/min)"() -> (w105:dbl)
      n42 = local read "Sample name:"() -> (w112:string)
      n43 = local read "Notes:"() -> (w114:string)
      n44 = Get Date/Time In Seconds() -> (seconds since 1Jan1904=w108:timestamp)
      n45 = Get Date/Time String(seconds (now)=w108) -> (date string=w110:string)  [unwired: 2 in, 1 out]
      n46 = Number To Fractional String(number=w105) -> (F-format string=w104:string)  [unwired: 3 in]
      n47 = Concatenate Strings("Date: ", w110, w106, "Sample name: ", w112, w106, "Notes: ", w114, w106, "Sweeprate: ", w104, w106) -> (w118:string)
      n48 = local read "Measurement File"() -> (w115:path)
      n49 = Open/Create/Replace File(file path (use dialog)=w115, error in=w103, operation (0:open)=4) -> (refnum out=w117:refnum<file>, error out=w119:errorcluster)  [unwired: 3 in, 1 out]
      "Messfile Refnum" <- w117
      n50 = Write to Text File(file (use dialog)=w117, text=w118, error in=w119) -> (error out=w102:errorcluster)  [unwired: 1 in, 2 out]
    }
    frame #2 {
      w121 = "\t"
      w123 = "\r"
      # "Erstellen der Spalten-\nbeschriftungen"
      n51 = local read "Messfile Refnum"() -> (w134:refnum<file>)
      n52 = Set File Position(refnum=w134, from (0:start)=1, error in=w127) -> (refnum out=w140:refnum<file>, error out=w142:errorcluster)  [unwired: 1 in]
      n53 = Concatenate Strings(w123, "B-Field Y/R", w121, "B-Field Z/phi", w121, "LI 1 Vx", w121, "LI 1 Vy", w121, "LI 2 Vx", w121, "LI 2 Vy", w121, "LI 3 Vx", w121, "LI 3 Vy", w121, "LI 4 Vx", w121, "LI 4 Vy", w121, "HP (V)", w121, w121, "AH C (pF)" ("string"), w121, "AH loss" ("string"), w121, "Tempsensor (Ohm)" ("string"), w121, "Timestamp", w123) -> (w141:string)
      n54 = Write to Text File(file (use dialog)=w140, text=w141, error in=w142) -> (refnum out=w144:refnum<file>, error out=w143:errorcluster)  [unwired: 1 in, 1 out]
      n55 = Flush File(refnum=w144, error in=w143) -> (error out=w126:errorcluster)  [unwired: 1 out]
    }
  }
  n56 = case shown="2" w54 {
    tunnel: w53 -> [w152 _ _]
    tunnel: w24 -> [w151 w158 w160]
    tunnel: "Y-Axis Communications Config" -> [w150 w153 w164]
    tunnel: [w148 w156 w164] -> w8
    tunnel: [w147 w157 w159] -> w32
    tunnel: w56 -> [w146 _ _]
    tunnel: w50 -> [_ w154 _]
    tunnel: w31 -> [_ _ w163]
    tunnel: w30 -> [_ _ w162]
    tunnel: w29 -> [_ _ w161]
    frame #0 {
      n57 = call <userlib>:"430_TCP_Open.vi"("IP Address"=w152, "TCP Port"=w146, "error in (no error)"=w151) -> ("connection ID"=w149:refnum<k5>, "error out"=w147:errorcluster)  [unwired: 3 in, 1 out]
      n58 = Bundle By Name(cluster=w150, "connection ID"=w149) -> (w148:T3)
    }
    frame #1 {
      n59 = call <userlib>:"430_RS232_Open.vi"("VISA resource name"=w154, "error in (no error)"=w158) -> ("VISA resource name out"=w155:refnum<visa-resource-name>, "error out"=w157:errorcluster)  [unwired: 5 in]
      n60 = Bundle By Name(cluster=w153, "Serial Port"=w155) -> (w156:T3)
    }
    frame #2 {
      n61 = case shown="0, Default" w161 {
        tunnel: w162 -> [w168 _]
        tunnel: w163 -> [w167 _]
        tunnel: w160 -> [w166 w169]
        tunnel: [w165 w169] -> w159
        frame #0 {
          n62 = DevClear(2:w166, 3:w167, 4:w168) -> (0:w165:errorcluster)  [unwired: 1 out]
        }
        frame #1 {
        }
      }
    }
  }
  n63 = case shown="2" w55 {
    tunnel: w52 -> [w176 _ _]
    tunnel: w32 -> [w175 w182 w184]
    tunnel: [w174 w181 w183] -> w49
    tunnel: "Z-Axis Communications Config" -> [w173 w179 w188]
    tunnel: [w171 w180 w188] -> w9
    tunnel: w56 -> [w170 _ _]
    tunnel: w51 -> [_ w177 _]
    tunnel: w35 -> [_ _ w187]
    tunnel: w34 -> [_ _ w186]
    tunnel: w33 -> [_ _ w185]
    frame #0 {
      n64 = call <userlib>:"430_TCP_Open.vi"("IP Address"=w176, "TCP Port"=w170, "error in (no error)"=w175) -> ("connection ID"=w172:refnum<k5>, "error out"=w174:errorcluster)  [unwired: 3 in, 1 out]
      n65 = Bundle By Name(cluster=w173, "connection ID"=w172) -> (w171:T3)
    }
    frame #1 {
      n66 = call <userlib>:"430_RS232_Open.vi"("VISA resource name"=w177, "error in (no error)"=w182) -> ("VISA resource name out"=w178:refnum<visa-resource-name>, "error out"=w181:errorcluster)  [unwired: 5 in]
      n67 = Bundle By Name(cluster=w179, "Serial Port"=w178) -> (w180:T3)
    }
    frame #2 {
      n68 = case shown="0, Default" w187 {
        tunnel: w186 -> [w192 _]
        tunnel: w185 -> [w191 _]
        tunnel: w184 -> [w190 w193]
        tunnel: [w189 w193] -> w183
        frame #0 {
          n69 = DevClear(2:w190, 3:w191, 4:w192) -> (0:w189:errorcluster)  [unwired: 1 out]
        }
        frame #1 {
        }
      }
    }
  }
  n70 = call <userlib>:"Init YZ 2D.vi"("Max Ramp Rate Z-axis"="Max Ramp Rate - Z Axis (A/s)", "Max Ramp Rate Y-axis"="Max Ramp Rate - Y Axis (A/s)", "error in"=w49, "Z-Axis Communications Config"=w9, "Y-Axis Communications Config"=w8) -> ("error out"=w67:T5)  [unwired: 5 in]
  n71 = stacked-sequence {
    seq-local: [_ w201 _ _] -> [_ _ w248 _]
    seq-local: [_ w200 _ _] -> [_ _ w247 _]
    tunnel: w9 -> [_ w203 _ _]
    tunnel: w67 -> [_ w204 _ _]
    tunnel: [_ w199 _ _] -> w63
    tunnel: w8 -> [_ w202 _ _]
    frame #0 {
      n72 = case "Displays an open dialog for loading a file if desired." shown="True" "Prompt for File?" {
        frame #0 {
        }
        frame #1 {
          n73 = call-poly <vilib>:"Read From Spreadsheet File.vi"() -> ("all rows"=w198:dbl[][])  [unwired: 7 in, 4 out]
          n74 = Number To Fractional String(number=w198, precision (6)=i16 4) -> (F-format string=w197:string[][])  [unwired: 2 in]
          n75 = local write "Field Values"(w197) -> ()
        }
      }
      n76 = local write "Continue Execution?"(TRUE ("Continue Execution?")) -> ()
    }
    frame #1 {
      w212 = u16 3 items=["NEXT VECTOR", "RAMPING", "HOLDING", "PAUSE", "ZERO"] ("Ramping Control")
      n77 = call <userlib>:"Get Switch Present.vi"("error in"=w204, "Communications Config"=w202) -> ("error out"=w208:T5, "Switch Present?"=w209:bool)
      n78 = case shown="True" w209 {
        tunnel: w208 -> [w230 w239]
        tunnel: w202 -> [_ w232]
        tunnel: [0.0 w236] -> w200
        tunnel: [w230 w238] -> w207
        frame #0 {
        }
        frame #1 {
          n79 = call <userlib>:"Get Switch Heater Time.vi"("error in"=w239, "Communications Config"=w232) -> ("error out"=w235:T5, "Switch Heating Time (secs)"=w237:dbl)
          n80 = call <userlib>:"Get Switch Heater.vi"("error in"=w235, "Communications Config"=w232) -> ("error out"=w234:T5, "Switch Heater Indicator"=w233:bool)
          n81 = case shown="False" w233 {
            tunnel: [w244 w245] -> w238
            tunnel: w237 -> [w242 _]
            tunnel: [w242 0.0] -> w236
            tunnel: w234 -> [w240 w245]
            tunnel: w232 -> [w241 _]
            frame #0 {
              n82 = call <userlib>:"Set Switch Heater.vi"("error in"=w240, "Switch Heater Control"=TRUE, "Communications Config"=w241) -> ("error out"=w244:T5)
            }
            frame #1 {
            }
          }
        }
      }
      n83 = call <userlib>:"Get Switch Present.vi"("error in"=w207, "Communications Config"=w203) -> ("error out"=w205:T5, "Switch Present?"=w206:bool)
      n84 = case shown="True" w206 {
        tunnel: w205 -> [w213 w222]
        tunnel: w203 -> [_ w215]
        tunnel: [0.0 w219] -> w201
        tunnel: [w213 w221] -> w199
        frame #0 {
        }
        frame #1 {
          n85 = call <userlib>:"Get Switch Heater Time.vi"("error in"=w222, "Communications Config"=w215) -> ("error out"=w218:T5, "Switch Heating Time (secs)"=w220:dbl)
          n86 = call <userlib>:"Get Switch Heater.vi"("error in"=w218, "Communications Config"=w215) -> ("error out"=w217:T5, "Switch Heater Indicator"=w216:bool)
          n87 = case shown="False" w216 {
            tunnel: [w223 w228] -> w221
            tunnel: w220 -> [w226 _]
            tunnel: [w226 0.0] -> w219
            tunnel: w217 -> [w224 w228]
            tunnel: w215 -> [w225 _]
            frame #0 {
              n88 = call <userlib>:"Set Switch Heater.vi"("error in"=w224, "Switch Heater Control"=TRUE, "Communications Config"=w225) -> ("error out"=w223:T5)
            }
            frame #1 {
            }
          }
        }
      }
      n89 = local write "Ramping Control"(w212) -> ()
      n90 = local write "Switch Heaters"(TRUE ("Switch Heater Control")) -> ()
      n91 = property on="Switch Heaters" class="Boolean (strict)"("Disabled"=u8 1 ("Write Attribute")) -> ()  [unwired: 2 in, 2 out]
    }
    frame #2 {
      n92 = Max & Min(x=w248, y=w247) -> (max(x,y)=w249:dbl)  [unwired: 1 out]
      n93 = local write "STATUS"("Heating switches..." ("STATUS")) -> ()
      n94 = Add(x=w249, y=2) -> (x+y=w253:dbl)
      n95 = property on="Ramping Control" class="Ring (strict)"("Disabled"=u8 1 ("Write Attribute")) -> ()  [unwired: 2 in, 2 out]
      n96 = Multiply(x=w253, y=1000) -> (x*y=w252:dbl)
      n97 = Wait (ms)(milliseconds to wait=w252) -> ()  [unwired: 1 out]
    }
    frame #3 {
      n98 = property on="Ramping Control" class="Ring (strict)"("Disabled"=u8 0 ("Write Attribute")) -> ()  [unwired: 2 in, 2 out]
      n99 = local write "STATUS"("Ready to ramp to first vector. Set Ramping Mode to NEXT VECTOR to begin." ("STATUS")) -> ()
      n100 = local read "Field Values"() -> (w258:string[][])
      n101 = Array Size(array=w258) -> (size(s)=w257:i32[])
      n102 = Index Array(array=w257, index=0) -> (element=→"Number of lines":i32)
    }
  }
  n103 = local read "Coordinate System"() -> (w64:u16)
  n104 = local read "Magnetic Field Units"() -> (w62:u16)
  n105 = Divide(x=180.0, y=3.141592653589793) -> (x/y=w59:dbl)
  n106 = while {
    shift-left: u16 6 ("Ramping Control") -> [w287]
    shift-right: [w288] -> _
    tunnel: [w290] -> w4
    tunnel: w9 -> [w264]
    tunnel: w8 -> [w265]
    tunnel: w59 -> [w292]
    tunnel: w62 -> [w293]
    tunnel: w63 -> [w294]
    tunnel: w9 -> [w295]
    tunnel: w8 -> [w296]
    tunnel: w64 -> [w282]
    tunnel: "Max Ramp Rate - Y Axis (A/s)" -> [w286]
    tunnel: "Max Ramp Rate - Z Axis (A/s)" -> [w285]
    tunnel: "Operation" -> [w284]
    tunnel: "LI 1" -> [w279]
    tunnel: "LI 2" -> [w278]
    tunnel: "LI 3" -> [w277]
    tunnel: "HP 1" -> [w276]
    tunnel: "HP 2" -> [w275]
    tunnel: "GPIB HP" -> [w274]
    tunnel: "GPIB HP 2" -> [w273]
    tunnel: "GPIB L 1" -> [w272]
    tunnel: "GPIB L 2" -> [w271]
    tunnel: "GPIB L 3" -> [w270]
    tunnel: "Nr. of Accumulations" -> [w269]
    shift-right: [w267] -> _
    shift-left: 0.0 -> [w266]
    tunnel: [w265] -> w5
    tunnel: [w264] -> w6
    tunnel: "AH (2500)" -> [w263]
    tunnel: "TempSensor" -> [w262]
    stop <- w289 continue-if-true
    n107 = stacked-sequence {
      seq-local: [w299 _] -> [_ w372]
      seq-local: [w298 _] -> [_ w369]
      tunnel: w282 -> [w305 _]
      tunnel: w296 -> [w304 _]
      tunnel: w295 -> [w303 _]
      tunnel: w294 -> [w302 _]
      tunnel: w293 -> [w301 _]
      tunnel: w292 -> [w300 _]
      tunnel: [_ w372] -> w283
      tunnel: [_ w369] -> w280
      tunnel: [w297 _] -> w281
      tunnel: [_ w370] -> w267
      tunnel: w266 -> [_ w371]
      frame #0 {
        # "Read B Field"
        n108 = case shown="1" w305 {
          tunnel: w304 -> [w315 w339]
          tunnel: w303 -> [w314 w338]
          tunnel: w302 -> [w313 w337]
          tunnel: w301 -> [w312 w336]
          tunnel: w300 -> [_ w335]
          tunnel: [w308 w334] -> w299
          tunnel: [w307 w332] -> w298
          tunnel: [w306 w333] -> w297
          tunnel: [_ w331] -> _
          frame #0 {
            n109 = call <userlib>:"Get 2D Field (Cartesian).vi"("Y-Axis Communications Config"=w315, "Z-Axis Communications Config"=w314, "error in"=w313) -> ("All Instruments Responded?"=w309:bool, "Y-Axis Field (kG)"=w311:dbl, "Z-Axis Field (kG)"=w310:dbl, "error out"=w308:T5)  [unwired: 2 in]
            n110 = case shown="1" w312 {
              tunnel: w311 -> [w316 w324]
              tunnel: w310 -> [w317 w325]
              tunnel: w309 -> [w318 w327]
              tunnel: [w317 w323] -> w307
              tunnel: [w316 w322] -> w306
              frame #0 {
                n111 = case shown="True" w318 {
                  tunnel: w316 -> [_ w320]
                  tunnel: w317 -> [_ w319]
                  frame #0 {
                  }
                  frame #1 {
                    n112 = Bundle("Y-Axis Field (kG)"=w320, "Z-Axis Field (kG)"=w319) -> (→"Cartesian Display (kG)":T6)  [unwired: 1 in]
                  }
                }
              }
              frame #1 {
                w326 = 0.1 ("y")
                n113 = Multiply(x=w324, y=w326) -> (x*y=w322:dbl)
                n114 = Multiply(x=w325, y=w326) -> (x*y=w323:dbl)
                n115 = case shown="True" w327 {
                  tunnel: w322 -> [_ w330]
                  tunnel: w323 -> [_ w329]
                  frame #0 {
                  }
                  frame #1 {
                    n116 = Bundle(w330, w329) -> (→"Cartesian Display (T)":cluster{dbl, dbl})  [unwired: 1 in]
                  }
                }
              }
            }
          }
          frame #1 {
            n117 = stacked-sequence {
              tunnel: w339 -> [w350]
              tunnel: w338 -> [w349]
              tunnel: w337 -> [w348]
              tunnel: w336 -> [w347]
              tunnel: w335 -> [w344]
              tunnel: [w342] -> w334
              tunnel: [w340] -> w332
              tunnel: [w341] -> w333
              tunnel: [w340] -> w331
              frame #0 {
                # "Field"
                n118 = call <userlib>:"Get 2D Field (Polar).vi"("Y-Axis Communications Config"=w350, "Z-Axis Communications Config"=w349, "error in"=w348) -> ("All Instruments Responded?"=w343:bool, "Radial (r) Field (kG)"=w346:dbl, "q (radians)"=w345:dbl, "error out"=w342:T5)  [unwired: 2 in]
                n119 = case shown="1" w347 {
                  tunnel: w346 -> [w352 w364]
                  tunnel: w345 -> [w354 w363]
                  tunnel: w344 -> [w353 w362]
                  tunnel: w343 -> [w355 w361]
                  tunnel: [w351 w359] -> w340
                  tunnel: [w351 w360] -> w341
                  frame #0 {
                    n120 = Multiply(x=w354, y=w353) -> (x*y=w351:dbl)
                    n121 = case shown="False" w355 {
                      tunnel: w352 -> [_ w356]
                      tunnel: w351 -> [_ w357]
                      frame #0 {
                      }
                      frame #1 {
                        n122 = Bundle(w357, "Radial (r) Field (kG)"=w356) -> (→"Polar Display (kG)":cluster{dbl, "Radial (r) Field (kG)":dbl})  [unwired: 1 in]
                      }
                    }
                  }
                  frame #1 {
                    n123 = Multiply(x=w364, y=0.1) -> (x*y=w360:dbl)
                    n124 = Multiply(x=w363, y=w362) -> (x*y=w359:dbl)
                    n125 = case shown="True" w361 {
                      tunnel: w360 -> [_ w366]
                      tunnel: w359 -> [_ w367]
                      frame #0 {
                      }
                      frame #1 {
                        n126 = Bundle(w367, w366) -> (→"Polar Display (T)":cluster{dbl, dbl})  [unwired: 1 in]
                      }
                    }
                  }
                }
              }
            }
          }
        }
      }
      frame #1 {
        # "Change PID"
        n127 = case shown="False" "Change\nPID\n(polar coordinates)" {
          tunnel: w371 -> [_ w378]
          tunnel: [_ w374] -> w370
          tunnel: w369 -> [_ w374]
          frame #0 {
          }
          frame #1 {
            n128 = local read "fieldvalues"() -> (w375:string[])
            n129 = call "SIM960Control.vi"("New Angle"=w374, "Old angle"=w378) -> ()  [unwired: 10 in]
            n130 = Index Array(array=w375, index=1 ("Index")) -> (element=w376:string)
            n131 = Fract/Exp String To Number(string=w376) -> ()  [unwired: 3 in, 2 out]
          }
        }
      }
    }
    n132 = local read "Ramping Control"() -> (w291:u16)
    n133 = local read "Messfile Refnum"() -> (w268:refnum<file>)
    n134 = case shown="1" w291 {
      selector: w291 -> [w380 w413 w573 w577 w592]
      tunnel: w265 -> [_ w415 _ w580 w597]
      tunnel: w264 -> [_ w414 _ w579 w596]
      tunnel: [w379 w385 w572 w578 w595] -> w290
      tunnel: [w380 w413 w573 w577 w592] -> w288
      tunnel: w287 -> [_ _ _ w576 w594]
      tunnel: w286 -> [_ _ _ _ w591]
      tunnel: w285 -> [_ _ _ _ w590]
      tunnel: w284 -> [_ w405 _ _ _]
      tunnel: w283 -> [w379 w401 w572 w574 w589]
      tunnel: w281 -> [_ w398 _ _ _]
      tunnel: w280 -> [_ w397 _ _ _]
      tunnel: w279 -> [_ w396 _ _ _]
      tunnel: w278 -> [_ w395 _ _ _]
      tunnel: w277 -> [_ w394 _ _ _]
      tunnel: w276 -> [_ w393 _ _ _]
      tunnel: w275 -> [_ w392 _ _ _]
      tunnel: w274 -> [_ w391 _ _ _]
      tunnel: w273 -> [_ w390 _ _ _]
      tunnel: w272 -> [_ w389 _ _ _]
      tunnel: w271 -> [_ w388 _ _ _]
      tunnel: w270 -> [_ w387 _ _ _]
      tunnel: w269 -> [_ w384 _ _ _]
      tunnel: w268 -> [_ w383 _ _ _]
      tunnel: w263 -> [_ w382 _ _ _]
      tunnel: w262 -> [_ w381 _ _ _]
      frame #0 {
      }
      frame #1 {
        w408 = T9."HOLDING" ("y")
        n135 = local read "Number of lines"() -> (w402:i32)
        n136 = local read "Starting index"() -> (w404:i32)
        n137 = call <userlib>:"Get Ramping Mode.vi"("Communications Config"=w415, "error in"=w401) -> ("Ramping Mode"=w411:T10, "error out"=w412:T5)  [unwired: 1 out]
        n138 = call <userlib>:"Get Ramping Mode.vi"("Communications Config"=w414, "error in"=w412) -> ("Ramping Mode"=w410:T10, "error out"=w386:T5)  [unwired: 1 out]
        n139 = Less?(x=w404, y=w402) -> (x < y?=w403:bool)
        n140 = Equal?(x=w411, y=w408) -> (x = y?=w407:bool)
        n141 = Equal?(x=w410, y=w408) -> (x = y?=w406:bool)
        n142 = Compound Arithmetic op=AND(w407, w406) -> (w409:bool)
        n143 = case shown="True" w409 {
          tunnel: w405 -> [_ w438]
          tunnel: w403 -> [_ w437]
          tunnel: "Wait between \nVectors (ms)" -> [_ w436]
          tunnel: "Wait between \nVectors" -> [_ w435]
          tunnel: w398 -> [_ w434]
          tunnel: w397 -> [_ w433]
          tunnel: w396 -> [_ w432]
          tunnel: w395 -> [_ w431]
          tunnel: w394 -> [_ w430]
          tunnel: w393 -> [_ w429]
          tunnel: w392 -> [_ w428]
          tunnel: w391 -> [_ w427]
          tunnel: w390 -> [_ w426]
          tunnel: w389 -> [_ w425]
          tunnel: w388 -> [_ w424]
          tunnel: w387 -> [_ w423]
          tunnel: w386 -> [w416 w422]
          tunnel: [w416 w421] -> w385
          tunnel: w384 -> [_ w420]
          tunnel: w383 -> [_ w419]
          tunnel: w382 -> [_ w418]
          tunnel: w381 -> [_ w417]
          frame #0 {
          }
          frame #1 {
            n144 = case shown="1" w438 {
              tunnel: w437 -> [_ w462]
              tunnel: w436 -> [_ w461]
              tunnel: w435 -> [_ w460]
              tunnel: w434 -> [_ w459]
              tunnel: w433 -> [_ w458]
              tunnel: w432 -> [_ w457]
              tunnel: w431 -> [_ w456]
              tunnel: w430 -> [_ w455]
              tunnel: w429 -> [_ w454]
              tunnel: w428 -> [_ w453]
              tunnel: w427 -> [_ w452]
              tunnel: w426 -> [_ w451]
              tunnel: w425 -> [_ w450]
              tunnel: w424 -> [_ w449]
              tunnel: w423 -> [_ w448]
              tunnel: w422 -> [w439 w447]
              tunnel: [w439 w446] -> w421
              tunnel: w420 -> [_ w445]
              tunnel: w419 -> [_ w444]
              tunnel: w418 -> [_ w443]
              tunnel: w417 -> [_ w442]
              frame #0 {
                w441 = u16 2 items=["NEXT VECTOR", "RAMPING", "HOLDING", "PAUSE", "ZERO"] ("Ramping Control")
                n145 = local write "STATUS"("Holding at current vector. Set Ramping Mode to NEXT VECTOR to continue." ("STATUS")) -> ()
                n146 = local write "Ramping Control"(w441) -> ()
              }
              frame #1 {
                # "Go to NEXT VECTOR automatically"
                n147 = case shown="True" w462 {
                  tunnel: w461 -> [_ w486]
                  tunnel: w460 -> [_ w485]
                  tunnel: w459 -> [_ w484]
                  tunnel: w458 -> [_ w483]
                  tunnel: w457 -> [_ w482]
                  tunnel: w456 -> [_ w481]
                  tunnel: w455 -> [_ w480]
                  tunnel: w454 -> [_ w479]
                  tunnel: w453 -> [_ w478]
                  tunnel: w452 -> [_ w477]
                  tunnel: w451 -> [_ w476]
                  tunnel: w450 -> [_ w475]
                  tunnel: w449 -> [_ w474]
                  tunnel: w448 -> [_ w473]
                  tunnel: w447 -> [w464 w472]
                  tunnel: [w464 w471] -> w446
                  tunnel: w445 -> [_ w470]
                  tunnel: w444 -> [_ w469]
                  tunnel: w443 -> [_ w468]
                  tunnel: w442 -> [_ w467]
                  frame #0 {
                    w466 = u16 2 items=["NEXT VECTOR", "RAMPING", "HOLDING", "PAUSE", "ZERO"] ("Ramping Control")
                    n148 = local write "STATUS"("Holding at current vector. Set Ramping Mode to NEXT VECTOR to continue." ("STATUS")) -> ()
                    n149 = local write "Ramping Control"(w466) -> ()
                    n150 = local write "Continue Execution?"(FALSE) -> ()
                  }
                  frame #1 {
                    n151 = stacked-sequence {
                      tunnel: w486 -> [w506 _]
                      tunnel: w485 -> [w505 _]
                      tunnel: w484 -> [w504 _]
                      tunnel: w483 -> [w503 _]
                      tunnel: w482 -> [w502 _]
                      tunnel: w481 -> [w501 _]
                      tunnel: w480 -> [w500 _]
                      tunnel: w479 -> [w499 _]
                      tunnel: w478 -> [w498 _]
                      tunnel: w477 -> [w497 _]
                      tunnel: w476 -> [w496 _]
                      tunnel: w475 -> [w495 _]
                      tunnel: w474 -> [w494 _]
                      tunnel: w473 -> [w493 _]
                      tunnel: w472 -> [w492 _]
                      tunnel: [w491 _] -> w471
                      tunnel: w470 -> [w490 _]
                      tunnel: w469 -> [w489 _]
                      tunnel: w468 -> [w488 _]
                      tunnel: w467 -> [w487 _]
                      frame #0 {
                        n152 = case shown="True" w505 {
                          tunnel: w506 -> [_ w526]
                          tunnel: w504 -> [_ w525]
                          tunnel: w503 -> [_ w524]
                          tunnel: w502 -> [_ w523]
                          tunnel: w501 -> [_ w522]
                          tunnel: w500 -> [_ w521]
                          tunnel: w499 -> [_ w520]
                          tunnel: w498 -> [_ w519]
                          tunnel: w497 -> [_ w518]
                          tunnel: w496 -> [_ w517]
                          tunnel: w495 -> [_ w516]
                          tunnel: w494 -> [_ w515]
                          tunnel: w493 -> [_ w514]
                          tunnel: w492 -> [w507 w513]
                          tunnel: [w507 w512] -> w491
                          tunnel: w490 -> [_ w511]
                          tunnel: w489 -> [_ w510]
                          tunnel: w488 -> [_ w509]
                          tunnel: w487 -> [_ w508]
                          frame #0 {
                          }
                          frame #1 {
                            n153 = stacked-sequence {
                              tunnel: w526 -> [w527 _ _]
                              tunnel: w525 -> [_ w561 _]
                              tunnel: w524 -> [_ w560 _]
                              tunnel: [_ w530 _] -> _
                              tunnel: w523 -> [_ w559 _]
                              tunnel: w522 -> [_ w558 _]
                              tunnel: w521 -> [_ w557 _]
                              tunnel: w520 -> [_ w556 _]
                              tunnel: w519 -> [_ w555 _]
                              tunnel: w518 -> [_ w554 _]
                              tunnel: w517 -> [_ w553 _]
                              tunnel: w516 -> [_ w552 _]
                              tunnel: w515 -> [_ w551 _]
                              tunnel: w514 -> [_ w550 _]
                              tunnel: w513 -> [_ w549 _]
                              tunnel: [_ w534 _] -> w512
                              tunnel: w511 -> [_ w533 _]
                              tunnel: w510 -> [_ w530 _]
                              tunnel: w509 -> [_ w529 _]
                              tunnel: w508 -> [_ w528 _]
                              frame #0 {
                                n154 = Wait (ms)(milliseconds to wait=w527) -> ()  [unwired: 1 out]
                              }
                              frame #1 {
                                n155 = call "ReadallDevicesv2.vi"("GPIB HP 2"=w553, "HP 2"=w555, "AH"=w529, "GPIB HP"=w554, "HP 1"=w556, "error in"=w549, "LI 3"=w557, "GPIB L 3"=w550, "TempSensor"=w528, "LI 2"=w558, "GPIB L 2"=w551, "LI 1"=w559, "GPIB L 1"=w552, "Nr. of Accumulations"=w533, "Y-Axis Field (kG)"=w561, "Radial (r) Field (kG) 2"=w560) -> ("appended array"=w531:dbl[], "error out"=w535:errorcluster)  [unwired: 2 in]
                                "appended array" <- w531
                                n156 = Array To Spreadsheet String(array=w531, 3:"%.9f" ("format string")) -> (spreadsheet string=w536:string)  [unwired: 1 in]
                                n157 = local read "measured data"() -> (w548:dbl[][])
                                n158 = Insert Into Array(array=w548, new element=w531) -> (w532:dbl[][])  [unwired: 2 in]
                                n159 = Index Array(array=w532, index (col)="X Axis") -> (element=w547:dbl[])  [unwired: 1 in]
                                n160 = Index Array(array=w532, index (col)="Y Axis") -> (element=w546:dbl[])  [unwired: 1 in]
                                n161 = Set File Position(refnum=w530, from (0:start)=1, error in=w535) -> (refnum out=w541:refnum<file>, error out=w540:errorcluster)  [unwired: 1 in]
                                n162 = Bundle("measured data"=w547, "measured data"=w546) -> (w545:T2)  [unwired: 1 in]
                                n163 = local write "measured data"(w532) -> ()
                                n164 = Write to Text File(file (use dialog)=w541, text=w536, error in=w540) -> (refnum out=w538:refnum<file>, error out=w539:errorcluster)  [unwired: 1 in, 1 out]
                                n165 = local write "XY Graph"(w545) -> ()
                                n166 = Flush File(refnum=w538, error in=w539) -> (error out=w534:errorcluster)  [unwired: 1 out]
                              }
                              frame #2 {
                                # "Restart PID after PID logout"
                                n167 = local read "appended array"() -> (w567:dbl[])
                                n168 = Index Array(array=w567, index=10) -> (element=w565:dbl)
                                n169 = Absolute Value(x=w565) -> (abs(x)=w564:dbl)
                                n170 = Greater Or Equal?(x=w564, y=260.0) -> (x >= y?=w562:bool)
                                n171 = case shown="True" w562 {
                                frame #0 {
                                }
                                frame #1 {
                                n172 = call "SIM960restartPID.vi"("Restart Damping"=FALSE, "GPIB-Adress"="2") -> ()  [unwired: 10 in]
                                }
                                }
                              }
                            }
                          }
                        }
                      }
                      frame #1 {
                        w571 = u16 0 items=["NEXT VECTOR", "RAMPING", "HOLDING", "PAUSE", "ZERO"] ("Ramping Control")
                        n173 = local write "Ramping Control"(w571) -> ()
                        n174 = local write "STATUS"("Go to NEXT VECTOR" ("STATUS")) -> ()
                      }
                    }
                  }
                }
              }
            }
          }
        }
      }
      frame #2 {
      }
      frame #3 {
        n175 = Not Equal?(x=w577, y=w576) -> (x != y?=w575:bool)
        n176 = case shown="True" w575 {
          tunnel: w580 -> [_ w588]
          tunnel: w579 -> [_ w587]
          tunnel: [w581 w585] -> w578
          tunnel: w574 -> [w581 w582]
          frame #0 {
          }
          frame #1 {
            w583 = u16 1 items=["RAMP", "PAUSE", "MANUAL UP", "MANUAL DOWN", "ZERO"] ("Ramping Mode")
            n177 = call <userlib>:"Set Ramping Mode.vi"("error in"=w582, "Ramping Mode"=w583, "Communications Config"=w588) -> ("error out"=w586:T5)
            n178 = call <userlib>:"Set Ramping Mode.vi"("error in"=w586, "Ramping Mode"=w583, "Communications Config"=w587) -> ("error out"=w585:T5)
            n179 = local write "STATUS"("All Programmers are PAUSED. Set Ramping Mode to NEXT VECTOR to continue." ("STATUS")) -> ()
          }
        }
      }
      frame #4 {
        n180 = Not Equal?(x=w592, y=w594) -> (x != y?=w593:bool)
        n181 = case shown="True" w593 {
          tunnel: w597 -> [_ w606]
          tunnel: w596 -> [_ w605]
          tunnel: [w598 w601] -> w595
          tunnel: w591 -> [_ w604]
          tunnel: w590 -> [_ w603]
          tunnel: w589 -> [w598 w599]
          frame #0 {
          }
          frame #1 {
            w600 = u16 4 items=["RAMP", "PAUSE", "MANUAL UP", "MANUAL DOWN", "ZERO"] ("Ramping Mode")
            n182 = local write "STATUS"("Zeroing vector." ("STATUS")) -> ()
            n183 = call <userlib>:"Set Ramping Mode.vi"("error in"=w599, "Ramping Mode"=w600, "Communications Config"=w606) -> ("error out"=w609:T5)
            n184 = call <userlib>:"Set Ramping Mode.vi"("error in"=w609, "Ramping Mode"=w600, "Communications Config"=w605) -> ("error out"=w602:T5)
            n185 = call <userlib>:"Set Current Ramp Rate.vi"("Communications Config"=w606, "Ramp Rate (A/sec)"=w604, "error in"=w602) -> ("error out"=w607:T5)  [unwired: 2 in]
            n186 = call <userlib>:"Set Current Ramp Rate.vi"("Communications Config"=w605, "Ramp Rate (A/sec)"=w603, "error in"=w607) -> ("error out"=w601:T5)  [unwired: 2 in]
          }
        }
      }
    }
    n187 = local read "Continue Execution?"() -> (w289:bool)
  }
  n188 = local read "Magnetic Field Units"() -> (w65:u16)
  n189 = local read "Coordinate System"() -> (w66:u16)
  n190 = while {
    tunnel: "Starting index" -> [w617]
    tunnel: w9 -> [w623]
    tunnel: w8 -> [w624]
    tunnel: w65 -> [w625]
    tunnel: w66 -> [w626]
    tunnel: w63 -> [w629]
    tunnel: "Max Ramp Rate - Y Axis (A/s)" -> [w613]
    tunnel: "Max Ramp Rate - Z Axis (A/s)" -> [w612]
    tunnel: "Magnitude Limit (kG)" -> [w614]
    tunnel: "User defined Ramp Rate (T/min)" -> [w611]
    tunnel: "User defined Ramp Rate (T/min)" -> [w610]
    i -> [w616]
    stop <- w618 continue-if-true
    n191 = local read "Field Values"() -> (w620:string[][])
    n192 = Add(x=w617, y=w616) -> (x+y=w615:i32)
    n193 = while "Wait for NEXT VECTOR setting by operator." {
      tunnel: [w633] -> w628
      tunnel: w629 -> [w633]
      stop <- w634 continue-if-true
      w632 = u16 0 items=["NEXT VECTOR", "RAMPING", "HOLDING", "PAUSE", "ZERO"] ("Ramping Control")
      n194 = local read "Ramping Control"() -> (w635:u16)
      n195 = Not Equal?(x=w632, y=w635) -> (x != y?=w634:bool)
    }
    n196 = stacked-sequence {
      tunnel: w615 -> [w637 _ w643 _]
      frame #0 {
        (unwired) -2
        n197 = Subtract(x=w637, y=2) -> (x-y=w640:i32)
        n198 = Bundle(w640, -2) -> (w638:cluster{i32, i32})  [unwired: 1 in]
        n199 = property on="Field Values" class="Tbl (strict)"("Active Cell:Active Cell"=w638) -> ()  [unwired: 2 in, 2 out]
      }
      frame #1 {
        n200 = local read "Normal color"() -> (w641:u32)
        n201 = property on="Field Values" class="Tbl (strict)"("Active Cell:Cell Background Color"=w641) -> ()  [unwired: 2 in, 2 out]
      }
      frame #2 {
        n202 = Decrement(x=w643) -> (x-1=w642:i32)
        n203 = Bundle(w642, -2) -> (w645:cluster{i32, i32})  [unwired: 1 in]
        n204 = property on="Field Values" class="Tbl (strict)"("Active Cell:Active Cell"=w645) -> ()  [unwired: 2 in, 2 out]
      }
      frame #3 {
        n205 = property on="Field Values" class="Tbl (strict)"("Active Cell:Cell Background Color"="Highlight color") -> ()  [unwired: 2 in, 2 out]
      }
    }
    n206 = Index Array(array=w620, index (row)=w615) -> (element=w627:string[])  [unwired: 1 in]
    "fieldvalues" <- w627
    n207 = local write "Starting index"(w615) -> ()
    n208 = Add(x=1, y=w615) -> (x+y=w630:i32)
    n209 = Number To Decimal String(number=w630) -> (decimal integer string=w619:string)  [unwired: 1 in]
    n210 = stacked-sequence {
      tunnel: [_ w671] -> w621
      tunnel: [_ w670] -> w622
      tunnel: w628 -> [_ w666]
      tunnel: w627 -> [_ w665]
      tunnel: w626 -> [_ w664]
      tunnel: w625 -> [_ w663]
      tunnel: w624 -> [_ w662]
      tunnel: w623 -> [_ w661]
      tunnel: w619 -> [_ w660]
      tunnel: w614 -> [_ w658]
      tunnel: w613 -> [_ w657]
      tunnel: w612 -> [_ w652]
      tunnel: w611 -> [_ w656]
      tunnel: w610 -> [_ w655]
      frame #0 {
        w650 = u16 1 items=["NEXT VECTOR", "RAMPING", "HOLDING", "PAUSE", "ZERO"] ("Ramping Control")
        n211 = local write "Ramping Control"(w650) -> ()
      }
      frame #1 {
        n212 = call <userlib>:"Set 2D Next Vector_entwurf.vi"("Coordinate System"=w664, "Magnetic Field Units"=w663, 3:"User defined Ramp Rate (T/min)"=w655, "Magnitude Limit (kG)"=w658, "Y-Axis Communications Config"=w662, "Input Vector"=w665, "Z-Axis Communications Config"=w661, 10:"User defined Ramp Rate (T/min)"=w656, "Max Ramp Rate - Y Axis (A/s)"=w657, "error in"=w666, "Max Ramp Rate - Z Axis (A/s)"=w652) -> ("Y-Axis Ramp Rate (T/min)"=→"Current Ramp Rate Y (T/min)":dbl, "Within Limits?"=w671:bool, "Ramp Rate along Vector (T/min)"=→"Ramp Rate along Vector (T/min)":dbl, "Z-Axis Ramp Rate (T/min)"=→"Current Ramp Rate Z (T/min)":dbl, "All Instruments Responded?"=w670:bool, "error out"=w659:T5)  [unwired: 3 in]
        n213 = Concatenate Strings("Ramping to field vector " ("STATUS"), w660, "..." ("STATUS")) -> (w667:string)
        n214 = local write "error in"(w659) -> ()
        n215 = local write "STATUS"(w667) -> ()
      }
    }
    n216 = case shown="True" w621 {
      tunnel: w622 -> [_ w648]
      frame #0 {
        n217 = local write "STATUS"("Vector magnitude limt or maximum coil current exceeded. Vector ignored. VI halted." ("STATUS")) -> ()
      }
      frame #1 {
        n218 = case shown="True" w648 {
          frame #0 {
            n219 = local write "STATUS"("Not all programmers responded. VI halted." ("STATUS")) -> ()
          }
          frame #1 {
          }
        }
      }
    }
    n220 = Compound Arithmetic op=AND(w622, w621) -> (w618:bool)
    n221 = local write "Continue Execution?"(w618) -> ()
  }
  n222 = case shown="True" "go to zero at end of measurement" {
    tunnel: [w672 w676] -> w7
    tunnel: w6 -> [_ w675]
    tunnel: w5 -> [_ w674]
    tunnel: w4 -> [w672 w673]
    frame #0 {
      # "go to zero"
    }
    frame #1 {
      n223 = stacked-sequence {
        tunnel: w674 -> [w693]
        tunnel: w675 -> [w694]
        tunnel: w673 -> [w684]
        tunnel: [w683] -> _
        frame #0 {
          w688 = u16 0 items=["kG", "Tesla"] ("Magnetic Field Units")
          w689 = u16 0 items=["Cartesian", "Polar"] ("Coordinate System")
          n224 = Build Array("0", "0") -> (w690:string[])
          n225 = call <userlib>:"Set 2D Next Vector_entwurf.vi"("Coordinate System"=w689, "Magnetic Field Units"=w688, "Magnitude Limit (kG)"=45.0, "Y-Axis Communications Config"=w693, "Input Vector"=w690, "Z-Axis Communications Config"=w694, "User defined Ramp Rate (T/min)"=FALSE, "Max Ramp Rate - Y Axis (A/s)"=0.05, "error in"=w684, "Max Ramp Rate - Z Axis (A/s)"=0.15) -> ("error out"=w683:T5)  [unwired: 4 in, 5 out]
        }
      }
      n226 = local read "Magnetic Field Units"() -> (w678:u16)
      n227 = local read "Coordinate System"() -> (w679:u16)
      n228 = Divide(x=180.0, y=3.141592653589793) -> (x/y=w677:dbl)
      n229 = while {
        tunnel: w677 -> [w703]
        tunnel: w678 -> [w704]
        tunnel: w675 -> [w700]
        tunnel: w674 -> [w701]
        tunnel: [w702] -> _
        tunnel: w679 -> [w702]
        tunnel: [w697] -> w676
        tunnel: w673 -> [w696]
        stop <- w698 stop-if-true
        n230 = stacked-sequence {
          seq-local: [w746 _ _] -> [_ w837 _]
          seq-local: [w745 _ _] -> [_ w834 _]
          seq-local: [w743 _ _] -> [_ w835 _]
          seq-local: [_ w822 _] -> [_ _ w904]
          tunnel: w702 -> [w751 _ w902]
          tunnel: w701 -> [w750 _ _]
          tunnel: w700 -> [w749 _ _]
          tunnel: w704 -> [w748 _ _]
          tunnel: w703 -> [w747 _ _]
          tunnel: [_ w836 _] -> w699
          tunnel: w696 -> [w744 _ _]
          tunnel: [w743 _ _] -> _
          frame #0 {
            # "Read B Field"
            n231 = case shown="0, Default" w751 {
              tunnel: w750 -> [w761 w783]
              tunnel: w749 -> [w760 w782]
              tunnel: w748 -> [w759 w781]
              tunnel: w747 -> [_ w780]
              tunnel: [w755 w779] -> w746
              tunnel: [w754 w777] -> w745
              tunnel: [w753 w778] -> w743
              tunnel: w744 -> [w752 _]
              frame #0 {
                n232 = call <userlib>:"Get 2D Field (Cartesian).vi"("Y-Axis Communications Config"=w761, "Z-Axis Communications Config"=w760, "error in"=w752) -> ("All Instruments Responded?"=w756:bool, "Y-Axis Field (kG)"=w758:dbl, "Z-Axis Field (kG)"=w757:dbl, "error out"=w755:T5)  [unwired: 2 in]
                n233 = case shown="1" w759 {
                  tunnel: w758 -> [w762 w770]
                  tunnel: w757 -> [w763 w771]
                  tunnel: w756 -> [w764 w773]
                  tunnel: [w763 w769] -> w754
                  tunnel: [w762 w768] -> w753
                  frame #0 {
                    n234 = case shown="False" w764 {
                      tunnel: w762 -> [_ w767]
                      tunnel: w763 -> [_ w766]
                      frame #0 {
                      }
                      frame #1 {
                        n235 = Bundle("Y-Axis Field (kG)"=w767, "Z-Axis Field (kG)"=w766) -> (w765:T6)  [unwired: 1 in]
                        n236 = local write "Cartesian Display (kG)"(w765) -> ()
                      }
                    }
                  }
                  frame #1 {
                    w772 = 0.1 ("y")
                    n237 = Multiply(x=w770, y=w772) -> (x*y=w768:dbl)
                    n238 = Multiply(x=w771, y=w772) -> (x*y=w769:dbl)
                    n239 = case shown="True" w773 {
                      tunnel: w768 -> [_ w776]
                      tunnel: w769 -> [_ w775]
                      frame #0 {
                      }
                      frame #1 {
                        n240 = Bundle(w776, w775) -> (w774:cluster{dbl, dbl})  [unwired: 1 in]
                        n241 = local write "Cartesian Display (T)"(w774) -> ()
                      }
                    }
                  }
                }
              }
              frame #1 {
                n242 = stacked-sequence {
                  tunnel: w783 -> [w793]
                  tunnel: w782 -> [w792]
                  tunnel: w781 -> [w791]
                  tunnel: w780 -> [w788]
                  tunnel: [w786] -> w779
                  tunnel: [w785] -> w777
                  tunnel: [w784] -> w778
                  frame #0 {
                    # "Field"
                    n243 = call <userlib>:"Get 2D Field (Polar).vi"("Y-Axis Communications Config"=w793, "Z-Axis Communications Config"=w792) -> ("All Instruments Responded?"=w787:bool, "Radial (r) Field (kG)"=w790:dbl, "q (radians)"=w789:dbl, "error out"=w786:T5)  [unwired: 3 in]
                    n244 = case shown="1" w791 {
                      tunnel: w790 -> [w795 w807]
                      tunnel: w789 -> [w797 w806]
                      tunnel: w788 -> [w796 w805]
                      tunnel: w787 -> [w798 w804]
                      tunnel: [w795 w802] -> w785
                      tunnel: [w794 w803] -> w784
                      frame #0 {
                        n245 = Multiply(x=w797, y=w796) -> (x*y=w794:dbl)
                        n246 = case shown="True" w798 {
                          tunnel: w795 -> [_ w800]
                          tunnel: w794 -> [_ w801]
                          frame #0 {
                          }
                          frame #1 {
                            n247 = Bundle(w801, "Radial (r) Field (kG)"=w800) -> (w799:cluster{dbl, "Radial (r) Field (kG)":dbl})  [unwired: 1 in]
                            n248 = local write "Polar Display (kG)"(w799) -> ()
                          }
                        }
                      }
                      frame #1 {
                        n249 = Multiply(x=w807, y=0.1) -> (x*y=w803:dbl)
                        n250 = Multiply(x=w806, y=w805) -> (x*y=w802:dbl)
                        n251 = case shown="True" w804 {
                          tunnel: w803 -> [_ w810]
                          tunnel: w802 -> [_ w811]
                          frame #0 {
                          }
                          frame #1 {
                            n252 = Bundle(w811, w810) -> (w809:cluster{dbl, dbl})  [unwired: 1 in]
                            n253 = local write "Polar Display (T)"(w809) -> ()
                          }
                        }
                      }
                    }
                  }
                }
              }
            }
          }
          frame #1 {
            # "Zeile in Datei schreiben"
            # "Read and Save Devices"
            n254 = stacked-sequence {
              tunnel: [w840 _ _ _ _ _ _ _] -> w833
              tunnel: [w839 _ _ _ _ _ _ _] -> w832
              tunnel: [_ w853 _ _ _ _ _ _] -> w829
              tunnel: [_ w851 _ _ _ _ _ _] -> w828
              tunnel: [_ _ w863 _ _ _ _ _] -> w827
              tunnel: [_ _ w862 _ _ _ _ _] -> w826
              tunnel: [_ _ _ w874 _ _ _ _] -> w825
              tunnel: [_ _ _ 0.0 _ _ _ _] -> w824
              tunnel: [_ _ _ _ w880 _ _ _] -> w823
              tunnel: [_ _ _ _ _ _ _ w898] -> w813
              tunnel: [_ _ _ _ _ w886 _ _] -> w815
              tunnel: [_ _ _ _ _ w885 _ _] -> w814
              tunnel: [_ _ _ _ _ _ w892 _] -> w812
              frame #0 {
                n255 = local read "LI 1"() -> (w838:bool)
                n256 = case shown="False" w838 {
                  tunnel: ["0" ("Antwort2") w847] -> w842
                  tunnel: ["0" ("Antwort1") w846] -> w841
                  frame #0 {
                  }
                  frame #1 {
                    n257 = local read "GPIB L 1"() -> (w845:string)
                    n258 = call "LI-Ansteuerung.vi"("Frage2"="OUTP? 4", "Frage1"="OUTP? 1", "address string"=w845) -> ("Antwort2"=w847:string, "Antwort1"=w846:string)
                  }
                }
                n259 = Fract/Exp String To Number(string=w842) -> (number=w839:dbl)  [unwired: 3 in, 1 out]
                n260 = Fract/Exp String To Number(string=w841) -> (number=w840:dbl)  [unwired: 3 in, 1 out]
              }
              frame #1 {
                n261 = local read "LI 2"() -> (w850:bool)
                n262 = case shown="False" w850 {
                  tunnel: [w855 w858] -> w852
                  tunnel: [w855 w857] -> w854
                  frame #0 {
                    w855 = "0" ("Antwort1")
                  }
                  frame #1 {
                    n263 = local read "GPIB L 2"() -> (w856:string)
                    n264 = call "LI-Ansteuerung.vi"("Frage2"="OUTP? 4", "Frage1"="OUTP? 1", "address string"=w856) -> ("Antwort2"=w858:string, "Antwort1"=w857:string)
                  }
                }
                n265 = Fract/Exp String To Number(string=w852) -> (number=w851:dbl)  [unwired: 3 in, 1 out]
                n266 = Fract/Exp String To Number(string=w854) -> (number=w853:dbl)  [unwired: 3 in, 1 out]
              }
              frame #2 {
                n267 = local read "LI 3"() -> (w861:bool)
                n268 = case shown="False" w861 {
                  tunnel: [w866 w869] -> w864
                  tunnel: [w866 w868] -> w865
                  frame #0 {
                    w866 = "0" ("Antwort1")
                  }
                  frame #1 {
                    n269 = local read "GPIB L 3"() -> (w867:string)
                    n270 = call "LI-Ansteuerung.vi"("Frage2"="OUTP? 4", "Frage1"="OUTP? 1", "address string"=w867) -> ("Antwort2"=w869:string, "Antwort1"=w868:string)
                  }
                }
                n271 = Fract/Exp String To Number(string=w865) -> (number=w863:dbl)  [unwired: 3 in, 1 out]
                n272 = Fract/Exp String To Number(string=w864) -> (number=w862:dbl)  [unwired: 3 in, 1 out]
              }
              frame #3 {
                n273 = local read "HP 1"() -> (w872:bool)
                n274 = case shown="True" w872 {
                  tunnel: [0.0 ("Voltage") w877] -> w874
                  frame #0 {
                  }
                  frame #1 {
                    n275 = local read "GPIB HP"() -> (w876:string)
                    n276 = call "HP-ReadVoltagev2.vi"("String"="meas:volt:dc? 250,0.001", "HP-Mulitmeter\nGPIB Address"=w876) -> ("Voltage"=w877:dbl)  [unwired: 9 in]
                  }
                }
              }
              frame #4 {
                n277 = local read "HP 2"() -> (w879:bool)
                n278 = case shown="True" w879 {
                  tunnel: [0.0 ("Voltage") w884] -> w880
                  frame #0 {
                  }
                  frame #1 {
                    n279 = local read "GPIB HP 2"() -> (w882:string)
                    n280 = call "HP-ReadVoltagev2.vi"("String"="meas:volt:dc? 200,0.001", "HP-Mulitmeter\nGPIB Address"=w882) -> ("Voltage"=w884:dbl)  [unwired: 9 in]
                  }
                }
              }
              frame #5 {
                n281 = local read "AH (2500)"() -> (w887:bool)
                n282 = case shown="True" w887 {
                  tunnel: [w888 w890] -> w886
                  tunnel: [w888 w889] -> w885
                  frame #0 {
                    w888 = 0.0 ("Voltage")
                  }
                  frame #1 {
                    n283 = call "AHRead2550.vi"() -> ("loss"=w890:dbl, "capacitance"=w889:dbl)  [unwired: 9 in, 1 out]
                  }
                }
              }
              frame #6 {
                n284 = local read "TempSensor"() -> (w891:bool)
                n285 = case shown="True" w891 {
                  tunnel: [0.0 ("Voltage") w894] -> w892
                  frame #0 {
                  }
                  frame #1 {
                    n286 = call "Read_R_Bridge_new_v3.vi"("Port Num- TRBridge"="7", "GPIB-Adress"="2" ("GPIB SIM900")) -> ("R out"=w895:string)  [unwired: 8 in, 1 out]
                    n287 = Fract/Exp String To Number(string=w895) -> (number=w894:dbl)  [unwired: 3 in, 1 out]
                  }
                }
              }
              frame #7 {
                n288 = Get Date/Time In Seconds() -> (seconds since 1Jan1904=w899:timestamp)
                n289 = To Double Precision Float(number=w899) -> (double precision float=w898:dbl)
              }
            }
            n290 = Build Array(w835, w834, w833, w832, w829, w828, w826, w827, w825, w824, w823, w814, w815, w812, w813) -> (w822:dbl[])
            n291 = Array To Spreadsheet String(array=w822, 3:"%f" ("format string")) -> (spreadsheet string=w831:string)  [unwired: 1 in]
            n292 = local read "Messfile Refnum"() -> (w816:refnum<file>)
            n293 = Set File Position(refnum=w816, from (0:start)=1, error in=w837) -> (refnum out=w818:refnum<file>, error out=w819:errorcluster)  [unwired: 1 in]
            n294 = Write to Text File(file (use dialog)=w818, text=w831, error in=w819) -> (refnum out=w821:refnum<file>, error out=w820:errorcluster)  [unwired: 1 in, 1 out]
            n295 = Flush File(refnum=w821, error in=w820) -> (error out=w836:errorcluster)  [unwired: 1 out]
          }
          frame #2 {
            n296 = local read "X Axis"() -> (w901:enum16{"B", "phi"})
            n297 = local read "Y Axis"() -> (w900:T1)
            n298 = local read "measured data"() -> (w905:dbl[][])
            n299 = Insert Into Array(array=w905, new element=w904) -> (w903:dbl[][])  [unwired: 2 in]
            n300 = case shown="0, Default" w902 {
              tunnel: w903 -> [w921 w935]
              tunnel: w900 -> [w923 w934]
              tunnel: w901 -> [w911 w933]
              frame #0 {
                n301 = Index Array(array=w921, index (col)=1 ("disabled index (col)")) -> (element=w916:dbl[])  [unwired: 1 in]
                n302 = Index Array(array=w921, index (col)=0 ("disabled index (col)")) -> (element=w915:dbl[])  [unwired: 1 in]
                n303 = Square(x=w916) -> (x^2=w918:dbl[])
                n304 = Square(x=w915) -> (x^2=w919:dbl[])
                n305 = Index Array(array=w921, index (col)=w923) -> (element=w910:dbl[])  [unwired: 1 in]
                n306 = Divide(x=w916, y=w915) -> (x/y=w907:dbl[])
                n307 = Add(x=w919, y=w918) -> (x+y=w917:dbl[])
                n308 = Inverse Tangent(1:w907) -> (0:w906:dbl[])
                n309 = Square Root(x=w917) -> (sqrt(x)=w908:dbl[])
                n310 = Divide(x=w906, y=3.141592653589793) -> (x/y=w913:dbl[])
                n311 = Multiply(x=w913, y=180) -> (x*y=w909:dbl[])
                n312 = case shown="\"phi\"" w911 {
                  tunnel: w910 -> [w926 w929]
                  tunnel: w909 -> [_ w928]
                  tunnel: w908 -> [w925 _]
                  frame #0 {
                    n313 = Bundle(w925, "measured data"=w926) -> (w924:cluster{dbl[], "measured data":dbl[]})  [unwired: 1 in]
                    n314 = local write "XY Graph"(w924) -> ()
                  }
                  frame #1 {
                    n315 = Bundle(w928, "measured data"=w929) -> (w927:cluster{dbl[], "measured data":dbl[]})  [unwired: 1 in]
                    n316 = local write "XY Graph"(w927) -> ()
                  }
                }
              }
              frame #1 {
                n317 = Index Array(array=w935, index (col)=w933) -> (element=w932:dbl[])  [unwired: 1 in]
                n318 = Index Array(array=w935, index (col)=w934) -> (element=w931:dbl[])  [unwired: 1 in]
                n319 = Bundle("measured data"=w932, "measured data"=w931) -> (w930:T2)  [unwired: 1 in]
                n320 = local write "XY Graph"(w930) -> ()
              }
            }
            n321 = local write "measured data"(w903) -> ()
          }
        }
        n322 = local read "Change\nPID\n(polar coordinates)"() -> (w695:bool)
        n323 = stacked-sequence {
          seq-local: [w706 _ _ _] -> [_ w717 w728 w738]
          seq-local: [w705 _ _ _] -> [_ _ w727 _]
          tunnel: w701 -> [w715 _ w730 _]
          tunnel: w700 -> [w714 _ w729 _]
          tunnel: w699 -> [w713 _ _ _]
          tunnel: [w706 _ _ _] -> w698
          tunnel: [_ _ w726 _] -> w697
          tunnel: w695 -> [_ w716 _ _]
          frame #0 {
            w709 = T9."HOLDING" ("y")
            n324 = call <userlib>:"Get Ramping Mode.vi"("Communications Config"=w715, "error in"=w713) -> ("Ramping Mode"=w711:T10, "error out"=w712:T5)  [unwired: 1 out]
            n325 = call <userlib>:"Get Ramping Mode.vi"("Communications Config"=w714, "error in"=w712) -> ("Ramping Mode"=w710:T10, "error out"=w705:T5)  [unwired: 1 out]
            n326 = Equal?(x=w710, y=w709) -> (x = y?=w708:bool)
            n327 = Equal?(x=w711, y=w709) -> (x = y?=w707:bool)
            n328 = And(x=w707, y=w708) -> (x .and. y?=w706:bool)
          }
          frame #1 {
            n329 = case shown="True" w717 {
              tunnel: w716 -> [_ w718]
              frame #0 {
              }
              frame #1 {
                n330 = case shown="True" w718 {
                  frame #0 {
                  }
                  frame #1 {
                    n331 = flat-sequence {
                      frame #0 {
                        n332 = call "SIM960Poff.vi"("off/on (0/1)"="0", "Port Num- PID"="1", "GPIB-Adress"="2") -> ()  [unwired: 9 in]
                      }
                      frame #1 {
                        n333 = call "SIM960Poff.vi"("off/on (0/1)"="0", "Port Num- PID"="3", "GPIB-Adress"="2") -> ()  [unwired: 9 in]
                      }
                    }
                  }
                }
                n334 = Wait (ms)(milliseconds to wait=u32 40000) -> ()  [unwired: 1 out]
              }
            }
          }
          frame #2 {
            n335 = case shown="True" w728 {
              tunnel: w730 -> [_ w737]
              tunnel: w729 -> [_ w736]
              tunnel: [w731 w733] -> w726
              tunnel: w727 -> [w731 w732]
              frame #0 {
              }
              frame #1 {
                w734 = u16 1 items=["RAMP", "PAUSE", "MANUAL UP", "MANUAL DOWN", "ZERO"] ("Ramping Mode")
                n336 = call <userlib>:"Set Ramping Mode.vi"("error in"=w732, "Ramping Mode"=w734, "Communications Config"=w737) -> ("error out"=w735:T5)
                n337 = call <userlib>:"Set Ramping Mode.vi"("error in"=w735, "Ramping Mode"=w734, "Communications Config"=w736) -> ("error out"=w733:T5)
              }
            }
          }
          frame #3 {
            n338 = case shown="True" w738 {
              frame #0 {
              }
              frame #1 {
                n339 = call <userlib>:"430_TCP_PSoff.vi"("IP Address"="111.111.111.2", "Switch Heater Control"=FALSE) -> ()  [unwired: 5 in, 2 out]
                n340 = call <userlib>:"430_TCP_PSoff.vi"("IP Address"="111.111.111.1", "Switch Heater Control"=FALSE) -> ()  [unwired: 5 in, 2 out]
              }
            }
          }
        }
      }
    }
  }
  n341 = Unbundle By Name(w9) -> ("Active Comm Interface"=w46:u16, "connection ID"=w45:refnum<k5>, "Serial Port"=w44:refnum<visa-resource-name>)
  n342 = Unbundle By Name(w8) -> ("Active Comm Interface"=w47:u16, "connection ID"=w43:refnum<k5>, "Serial Port"=w42:refnum<visa-resource-name>)
  n343 = case shown="0, Default" w47 {
    tunnel: w43 -> [w938 _ _]
    tunnel: [w937 w941 w942] -> w48
    tunnel: w42 -> [_ w940 _]
    tunnel: w7 -> [w936 w939 w942]
    frame #0 {
      n344 = call <userlib>:"430_TCP_Close.vi"("error in (no error)"=w936, "connection ID"=w938) -> ("error out"=w937:errorcluster)  [unwired: 1 out]
    }
    frame #1 {
      n345 = call <userlib>:"430_RS232_Close.vi"("error in (no error)"=w939, "VISA resource name"=w940) -> ("error out"=w941:errorcluster)  [unwired: 1 in]
    }
    frame #2 {
    }
  }
  n346 = case shown="0, Default" w46 {
    tunnel: w45 -> [w945 _ _]
    tunnel: w48 -> [w944 w948 w949]
    tunnel: [w943 w947 w949] -> w41
    tunnel: w44 -> [_ w946 _]
    frame #0 {
      n347 = call <userlib>:"430_TCP_Close.vi"("error in (no error)"=w944, "connection ID"=w945) -> ("error out"=w943:errorcluster)  [unwired: 1 out]
    }
    frame #1 {
      n348 = call <userlib>:"430_RS232_Close.vi"("error in (no error)"=w948, "VISA resource name"=w946) -> ("error out"=w947:errorcluster)  [unwired: 1 in]
    }
    frame #2 {
    }
  }
  "error out" <- w41
